vi "XY_plot_gnuplot.vi"(0 "Plot Array":cluster{dbl[], dbl[]}[](array[cluster])=[{[500.0, 500.0, 953.54, 215.0, 270.0, 320.0, 445.0, 525.0, 600.0, 675.0, 750.0, 825.0, 900.0, 960.0, 1010.0, 1060.0], [4.614524, 4.54365, 5.818368, 0.1374656, 0.6662545, 1.465458, 3.619824, 4.848976, 5.887329, 5.940571, 6.152151, 5.717487, 5.600293, 5.40069, 5.154843, 5.121789]}, {[100.0, 150.0, 215.0, 270.0, 320.0, 445.0, 525.0, 600.0, 675.0, 750.0, 825.0, 900.0, 960.0, 1010.0, 1060.0], [0.002314715, -0.00693192, 0.120417, 0.6880509, 1.519176, 3.513709, 5.065183, 6.116033, 6.096773, 5.938465, 5.593788, 5.5597, 5.387002, 5.304077, 4.887903]}] {"?" format="%.2f"; "?" format="%.2f"}, 1 "Job Directory":path=path "/G4_2_HD/Users/paulhayden/Documents/Projects/Westlakes_resolution") -> (2 "Saved Automatically?":bool, 3 "Tex Info String":string="set term epslatex\nset output \"Plot.eps\"\nset xlabel '$Distance~(m)$'\nset ylabel '$DF~(s/m^3)\\times10^6$'\nset samples 1000\nset pointsize 1.00\nset title '$B38~Centreline~Glc$' 0, 0\nset size 0.75,0.9\n\n#set key 450, -2.5833\n unset key\nset label 1 '~~~~~~~~~~~Angle~(deg)~=~0' at -100, -2.58\nset label 2 '~~~~~~~~~~~Height~(m)~=~5' at -100, -3.27\n set xrange [0 : 500] \n# set autoscale x \n set yrange [0.10000 : 7]\n# set autoscale y \n\nplot \"B38_Centreline_Glc.dat\" index 0 using 1:2 axes x1y1 title '$File=B38R~DDD.xls$' with points 1 1, \\\n\"B38_Centreline_Glc.dat\" index 1 using 1:2 axes x1y1 title '$File=B38R~DDD~1.xls$' with points 1 3", 4 "Plot data file":path)   [LabVIEW 2015]
uses:
  Gnuplot_Label.ctl
  gnuplotScriptComponents/gridlines.ctl
  gnuplotScriptComponents/legendAppearance.ctl
  gnuplotScriptComponents/legendProperties.ctl
  gnuplotScriptComponents/alignment.ctl
  gnuplotScriptComponents/at.ctl
  <vilib>/Analysis/baseanly.llb/Mean (DBL).vi
  Results_plotter_Global.vi
  <vilib>/Analysis/NI_AALBase.lvlib
  <vilib>/Analysis/NI_AALPro.lvlib
panel:
  in  "Current Fit Formula":string
  in  "Show Re-Run Gnuplot?":bool
  in  "Tab Control":T1(tab)
  in  "Plot Title":u16(ring) items=["Title String Only", "Stack::", "RunNum::", "WD::(deg)", "EBD::", "Stack:X:(mm ref TTC)", "User:Comments:", "Run:Messages:", "Exclude:Reason:", "X:Rel:(mm)", "Y:Rel:(mm)", "C:minusBG:(ppm)", "C:LatFit:Max(ppm)", "C:LatFit:SigmaY(mm)", "C:LatFit:Yo(mm)", "C:LatData:Max(ppm)", "Uref::(m/s)", "C:incBG:(ppm)", "C:Variance:(ppm^2)", "C:minusBG:(ppm)Err", "C:LatData:Max(ppm)Err", "BG:Conc:(ppm)", "BG:Variance:(ppm^2)", "BG:Conc:(ppm)Err", "FID:Num:", "FID:Calibration:Filename", "X:Trav:(mm)", "Y:Trav:(mm)", "Z (mm)::", "TrackedStack:Yat0deg:(mm)", "TrackedStack:Xat0deg:(mm)", "TrackedStack:Ycurrent:(mm)", "TrackedStack:Xcurrent:(mm)", "T::(C)", "P:Atm:(mbar)", "MFC:Enable:", "MFC24:Read:(%)", "MFC23:Read:(%)", "Date:of:Measurement", "Time:Measurement:Commenced", "Multi Run:Command:Filename", "Multi Run:Start Time:", "Multi Run:Row:Type", "Time:Stamp:(seconds)", "Original:Results:Filename", "Raw:Data:Filename", "EBD:Comments:", "EBD:Xdim:", "EBD:Ydim:", "EBD:Zdim:", "EBD:RunNum:", "EBD:X-Location:", "EBD:Y-Location:", "Number of Measurements"]
  in  "Plot Title":string
  in  "Added labels":i32[](listbox)
  in  "Show Labels?":bool
  in  "Summarise":u16(ring) items=["All Series", "EBD=0L\\times0W\\times0H @  0X, 0Y__Stack X (mm ref TTC)=Show All__", "EBD=80L\\times160W\\times80H @  -80X, 0Y__Stack X (mm ref TTC)=Show All__", "EBD=80L\\times160W\\times80H @  0X, 0Y__Stack X (mm ref TTC)=Show All__", "EBD=90L\\times180W\\times90H @  0X, 0Y__Stack X (mm ref TTC)=Show All__", "EBD=100L\\times200W\\times100H @  -100X, 0Y__Stack X (mm ref TTC)=Show All__"]
  in  "X Log?":bool
  in  "Y Log?":bool
  in  "Ymin Val":dbl
  in  "Ymin":bool=TRUE
  in  "Xmin Val":dbl
  in  "Xmin":bool=TRUE
  in  "Xmax Val":dbl
  in  "Xmax":bool=TRUE
  in  "Ymax Val":dbl
  in  "Ymax":bool=TRUE
  in  "Major Gridlines":T2
  in  "Minor Gridlines":T2
  out "Time format?":bool
  in  "precision":string
  out "Profile offset":dbl
  in  "Offset?":bool
  in  "Mode":T3
  in  "Separation":dbl=1.2
  in  "Fit Line Width":i32=2
  in  "Fit type":T4(ring)
  in  "Put Coeff\nin Results file":bool
  in  "Analysis":T5(ring)
  in  "Wavelength?":bool
  in  "Auto Zp":bool=TRUE
  in  "Fixed Zp":dbl format="%.2f"
  in  "Something about fit..!":bool
  in  "Fit Line Type":i32=2
  in  "Black and white?":bool
  in  "plot error bars?":bool
  in  "Plot style":u16[](array[ring])=[0, 0, 0, 0, 0, 0, 0, 0, 0, 0, 0] items=["points", "lines", "linespoints"]
  in  "Point Size":dbl=1.2 format="%.2f"
  in  "Graph Height":string="0.9"
  in  "Graph width":string="0.75"
  in  "Reverse order":bool
  in  "Appearance":T6
  in  "Show legend?":bool
  in  "Legend Position":u16(ring) items=["LabVIEW calculated", "top left", "top right", "bottom left", "bottom right", "below"]
  in  "Save data analysis file":bool
  out "Path":path
  in  "Filename Max length":i32=28
  out "With legend":i32=580
  out "No Legend":i32=397
  out "No of Series":i32=2
  out "X location":dbl=-100.0
  out "Y location":dbl=-2.583333333333333
  out "Delta y":dbl=0.6900000000000001
  out "Extra range":dbl
  out "Final Title":string="B38 Centreline Glc"
  out "XY Graph":cluster{dbl[], dbl[]}[](graph)=[{[215.0, 270.0, 320.0, 445.0, 500.0, 500.0, 525.0, 600.0, 675.0, 750.0, 825.0, 900.0, 953.54, 960.0, 1010.0, 1060.0], [0.1374656, 0.6662545, 1.465458, 3.619824, 4.614524, 4.54365, 4.848976, 5.887329, 5.940571, 6.152151, 5.717487, 5.600293, 5.818368, 5.40069, 5.154843, 5.121789]}, {[100.0, 150.0, 215.0, 270.0, 320.0, 445.0, 525.0, 600.0, 675.0, 750.0, 825.0, 900.0, 960.0, 1010.0, 1060.0], [0.002314715, -0.00693192, 0.120417, 0.6880509, 1.519176, 3.513709, 5.065183, 6.116033, 6.096773, 5.938465, 5.593788, 5.5597, 5.387002, 5.304077, 4.887903]}]
  # "Scales"
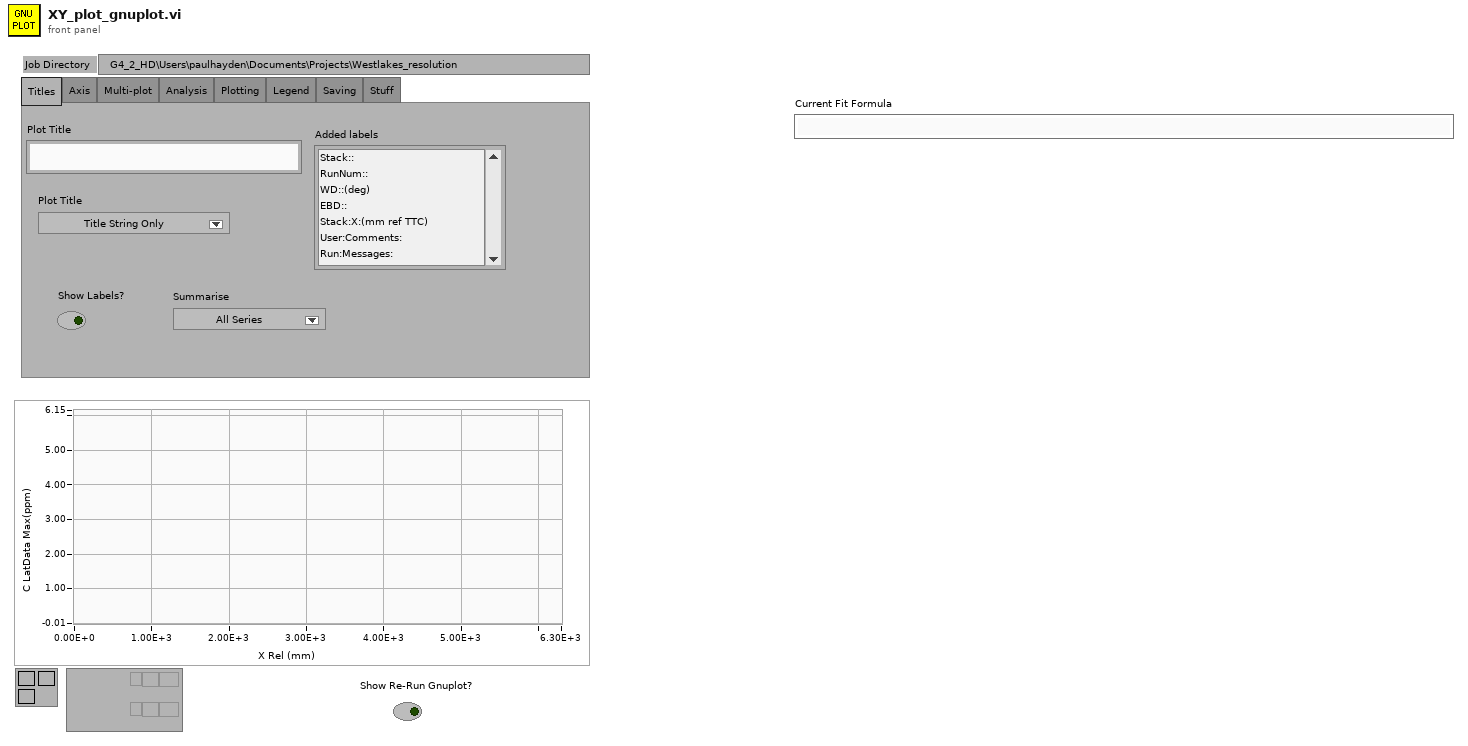
[diagram p1: front panel]
types:
  T1 = enum32{"Titles", "Axis", "Multi-plot", "Analysis", "Plotting", "Legend", "Saving", "Stuff"}
  T2 = typedef "gridlines.ctl" = enum16{"None", "X only", "Y only", "Both X and Y"}
  T3 = typedef "Gnuplot_Label.ctl" = enum16{"3 Labels per plot", "Only Center label", "Only Bottom Label"}
  T4 = enum16{"None", "Spline", "Linear", "2nd Poly", "3rd Poly", "4th Poly", "Gauss Lat", "Gauss vert", "Gauss Vert with 2 sig", "Guass glc"}
  T5 = enum16{"None", "% change", "Spectrum", "Norm Spec"}
  T6 = typedef "legendAppearance.ctl" = cluster{"layout":string, "text-sample order":string, "key order":string, "surroundingBox":string, "MaxRows":u32, "MaxCols":u32, "WidthAdjust":dbl}
  T7 = cluster{"Output":dbl[], "PercentageDifferenceArray":dbl[]}[]
  T8 = cluster{"Output":dbl[], "PercentageDifferenceArray":dbl[]}
  T9 = typedef "legendProperties.ctl" = cluster{"Appearance":T6, "Alignment":T10, "Location":string, "\"At\" location":T11}
  T10 = typedef "alignment.ctl" = cluster{"Horizontal":string, "Vertical":string}
  T11 = typedef "at.ctl" = cluster{"XcoordSys":string, "YcoordSys":string, "Xvalue":dbl, "Yvalue":dbl}
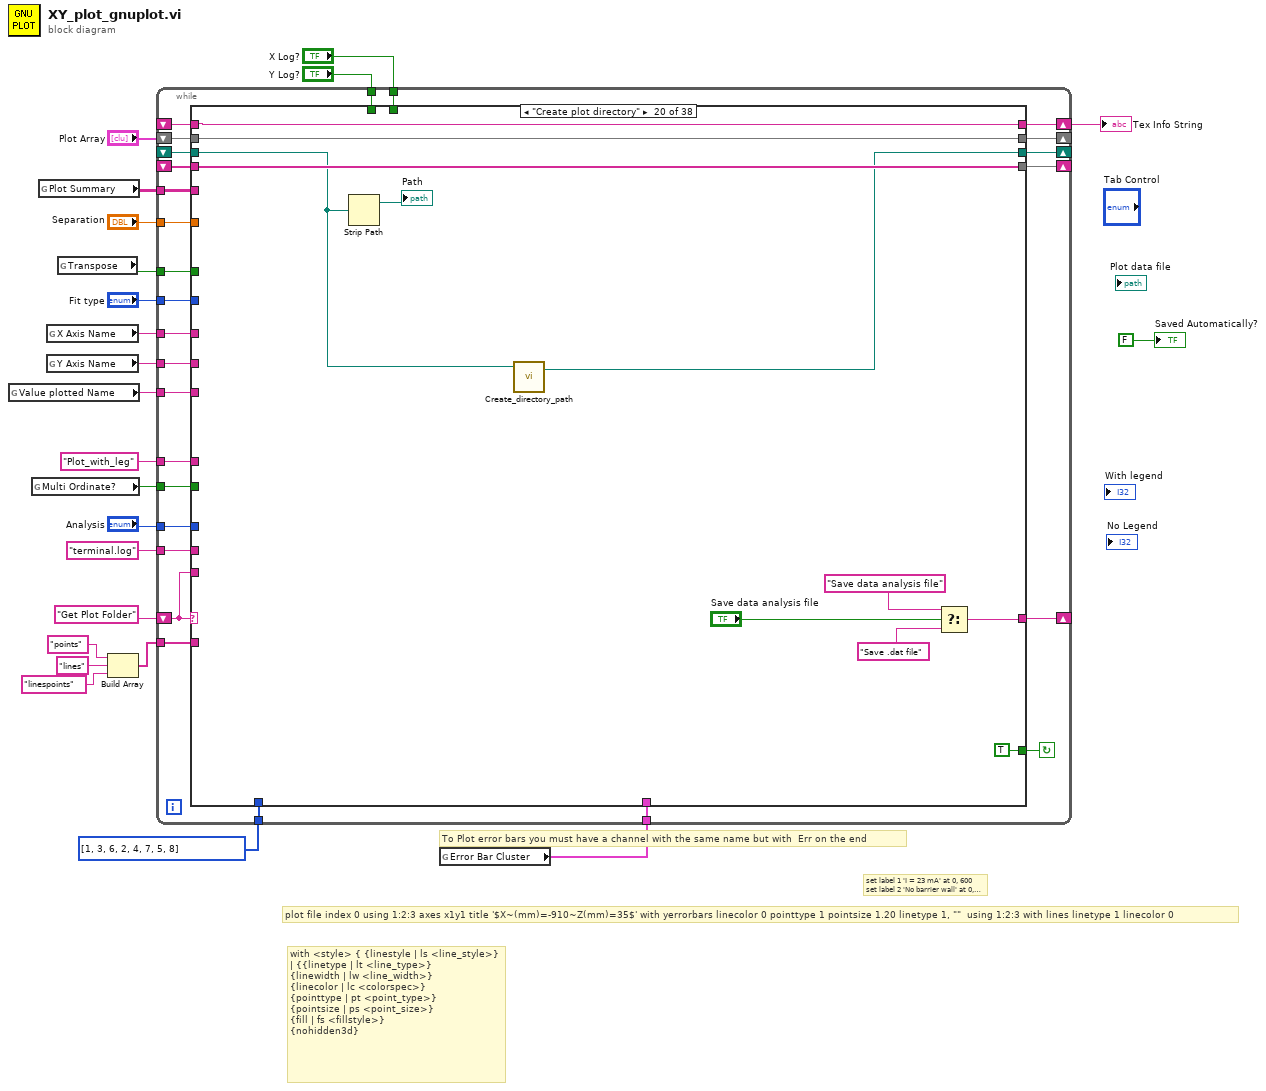
[diagram p0: block diagram]
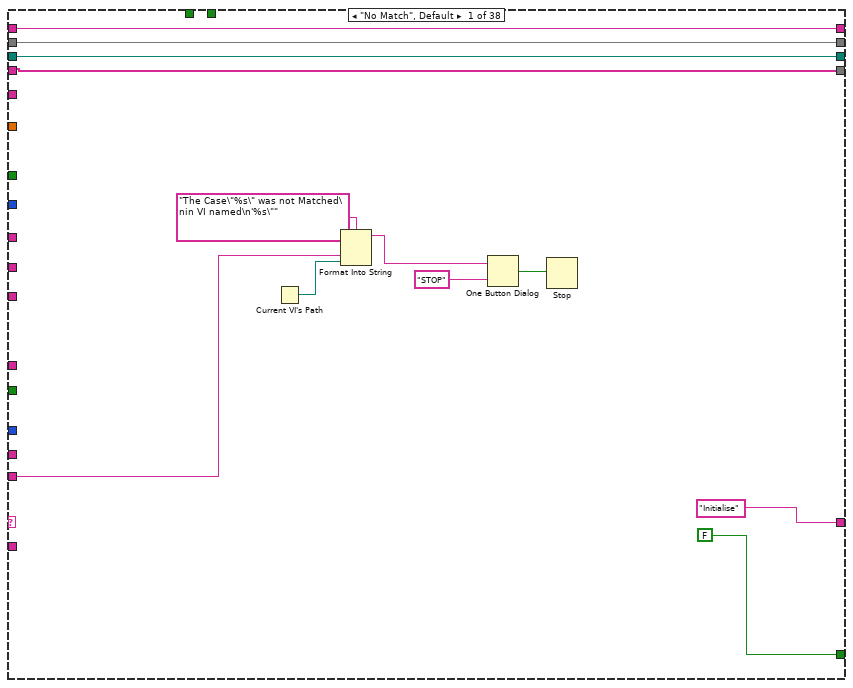
[diagram p2: hidden frame]
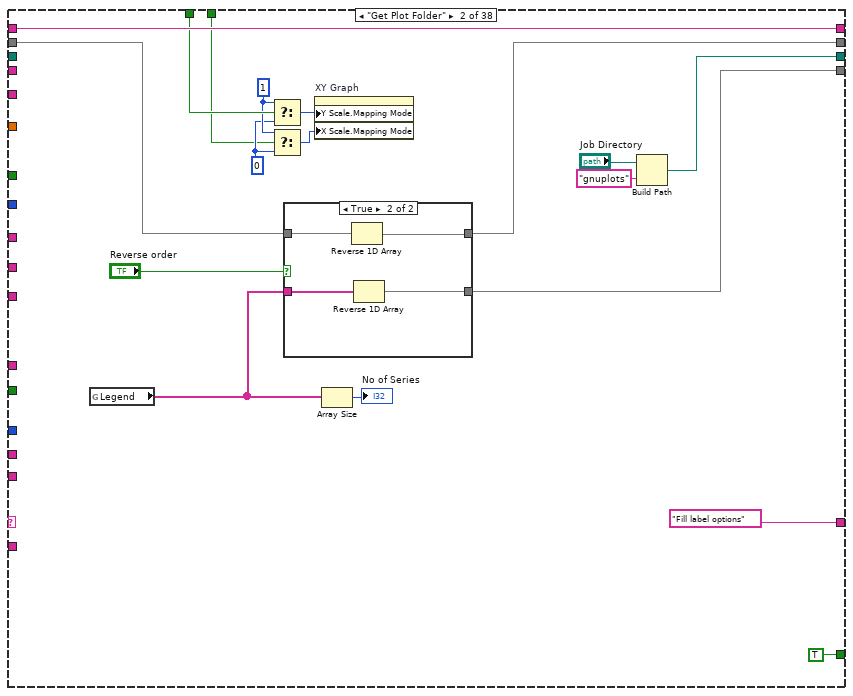
[diagram p3: hidden frame]
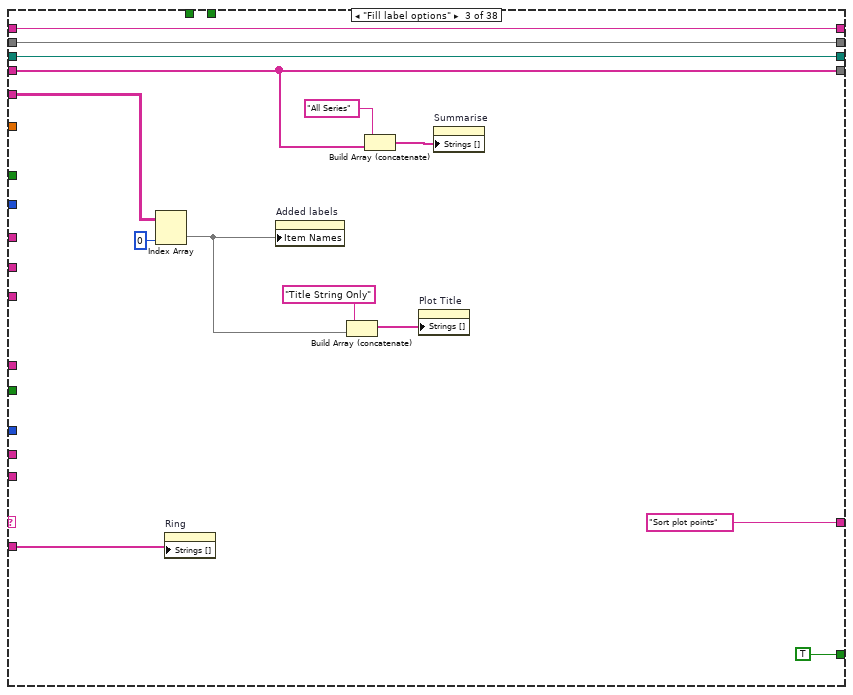
[diagram p5: hidden frame]
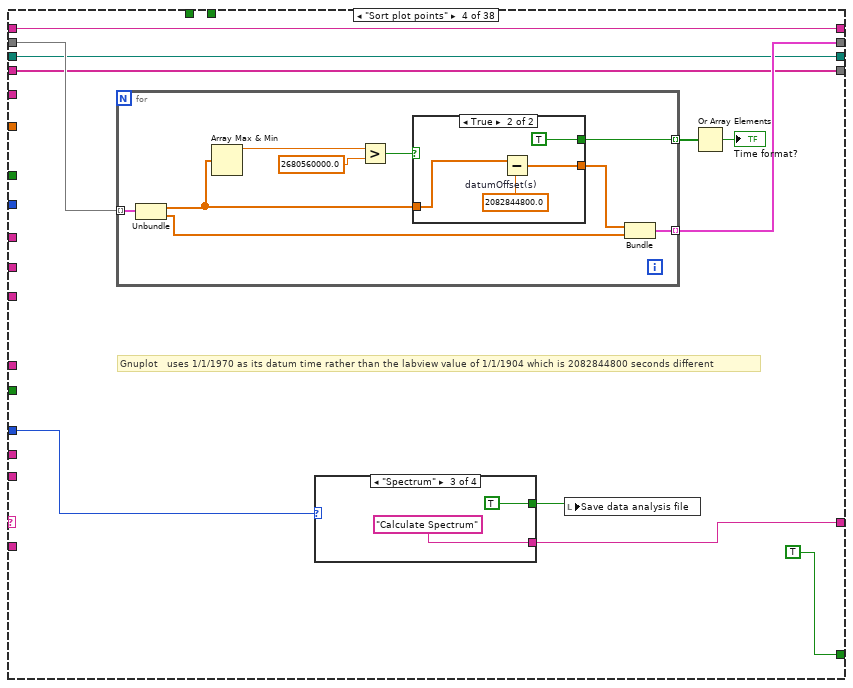
[diagram p6: hidden frame]
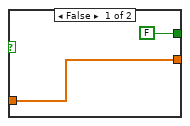
[diagram p7: hidden frame]
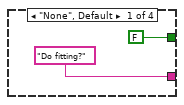
[diagram p8: hidden frame]
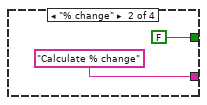
[diagram p9: hidden frame]
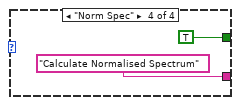
[diagram p10: hidden frame]
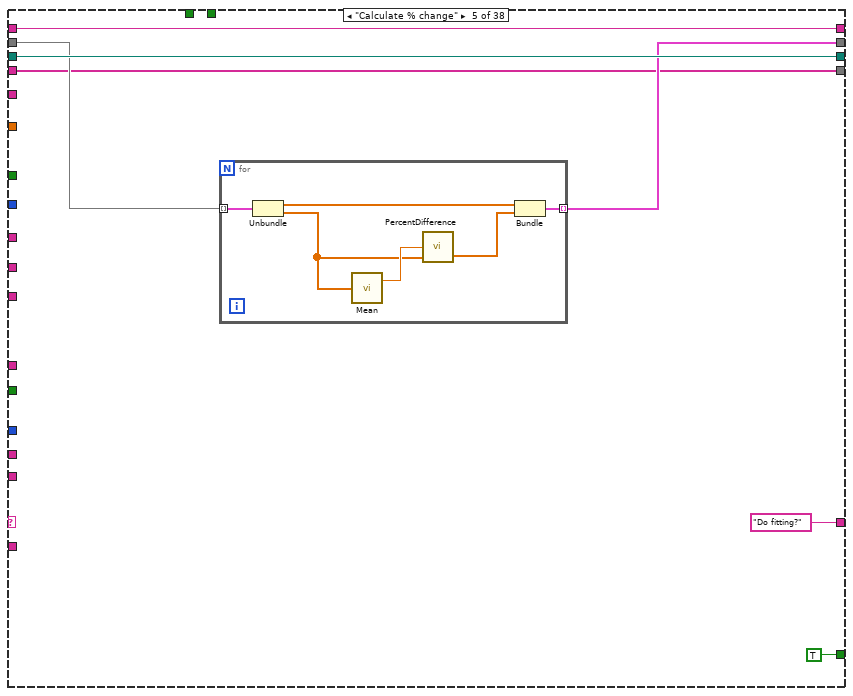
[diagram p11: hidden frame]
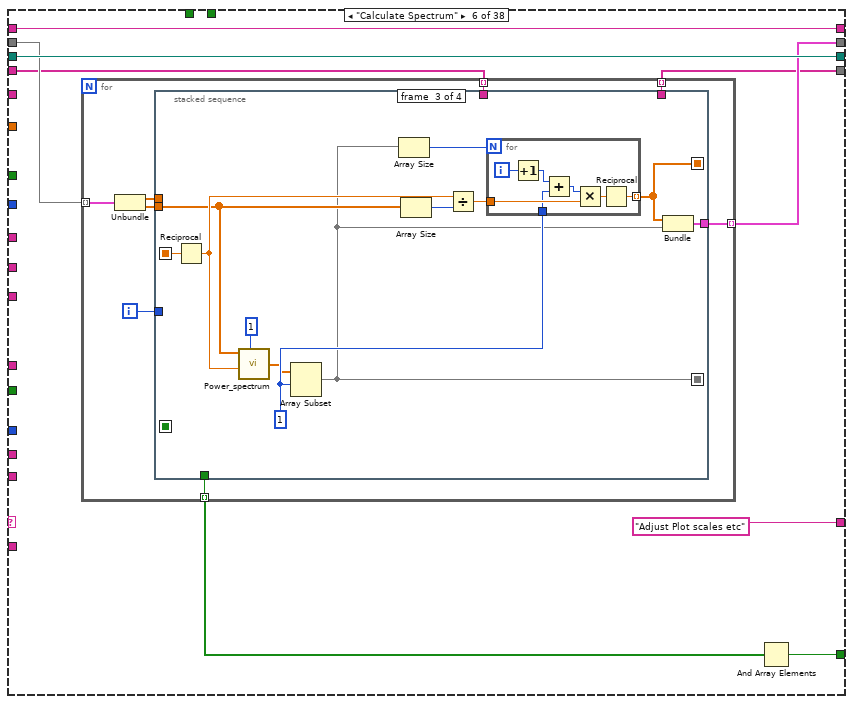
[diagram p12: hidden frame]
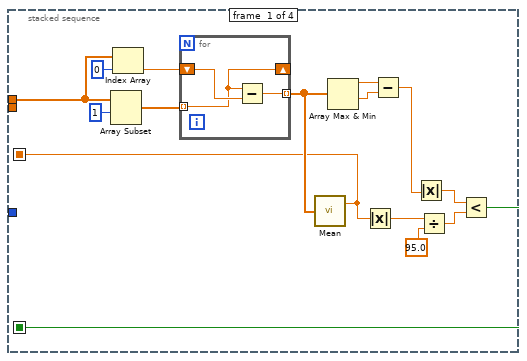
[diagram p13: hidden frame]
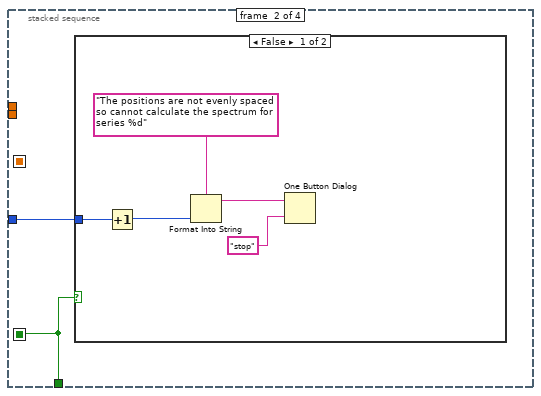
[diagram p14: hidden frame]
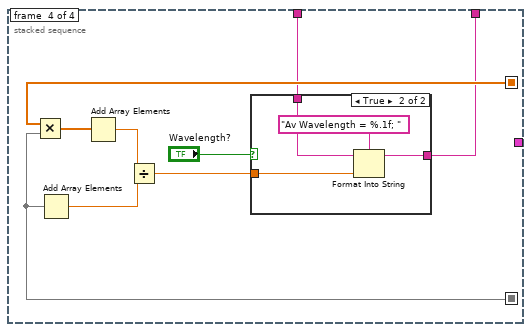
[diagram p16: hidden frame]
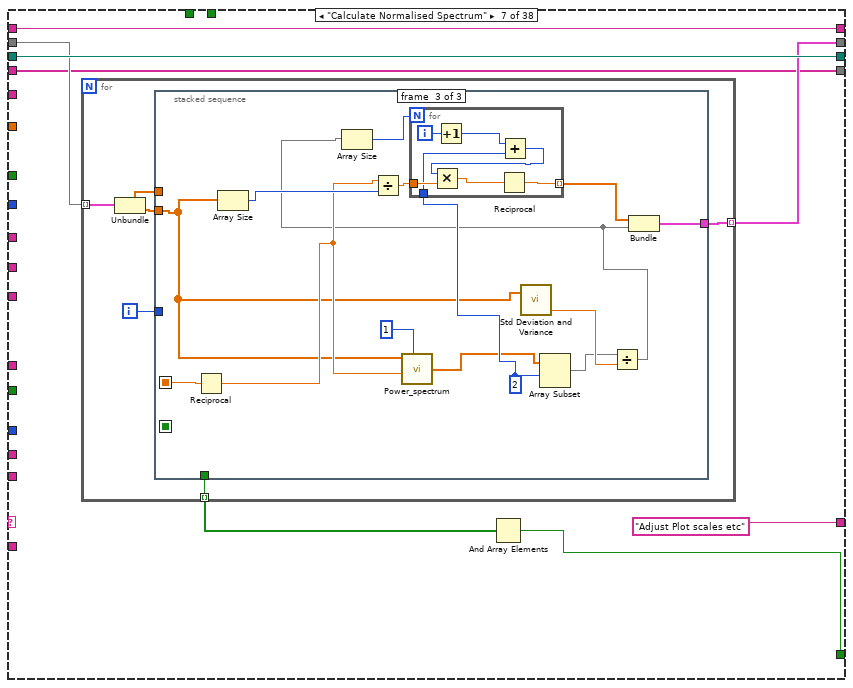
[diagram p18: hidden frame]
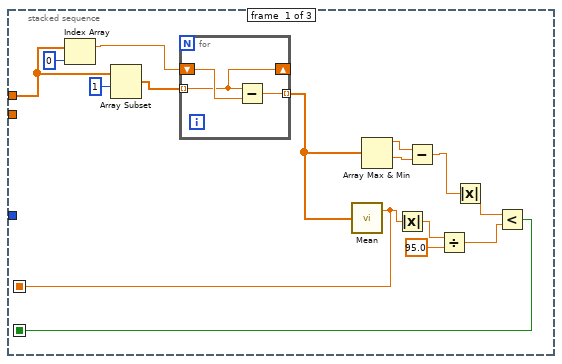
[diagram p19: hidden frame]
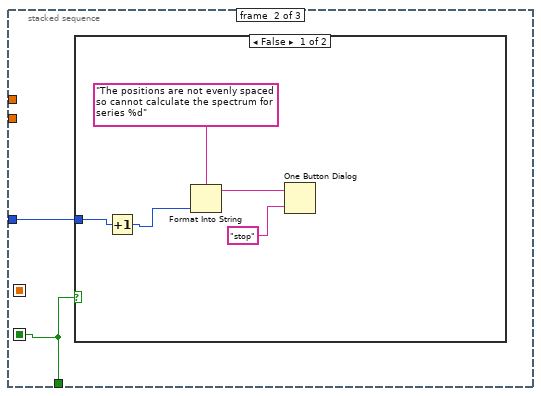
[diagram p20: hidden frame]
diagram:
  # "plot file index 0 using 1:2:3 axes x1y1 title '$X~(mm)=-910~Z(mm)=35$' with yerrorbars linecolor 0 pointtype 1 pointsize 1.20 linetype 1, \"\"  using 1:2:3 with lines linetype 1 linecolor 0"
  # "with <style> { {linestyle | ls <line_style>} \n| {{linetype | lt <line_type>} \n{linewidth | lw <line_width>} \n{linecolor | lc <colorspec>} \n{pointtype | pt <point_type>} \n{pointsize | ps <point_size>} \n{fill | fs <fillstyle>} \n{nohidden3d}"
  # "To Plot error bars you must have a channel with the same name but with  Err on the end"
  # "set label 1 'I = 23 mA' at 0, 600\nset label 2 'No barrier wall' at 0, 300"
  n1 = global read "Results_plotter_Global.vi" "Value plotted Name"() -> (w19:string)
  n2 = global read "Results_plotter_Global.vi" "Multi Ordinate?"() -> (w1:bool)
  n3 = global read "Results_plotter_Global.vi" "Plot Summary"() -> (w22:string[][])
  n4 = global read "Results_plotter_Global.vi" "X Axis Name"() -> (w21:string)
  n5 = global read "Results_plotter_Global.vi" "Y Axis Name"() -> (w20:string)
  n6 = global read "Results_plotter_Global.vi" "Transpose"() -> (w2:bool)
  n7 = Build Array("points", "lines", "linespoints") -> (w9:string[])
  n8 = global read "Results_plotter_Global.vi" "Error Bar Cluster"() -> (w4:cluster{string[]}[])
  n9 = while {
    shift-left: "Get Plot Folder" -> [w48]
    shift-right: [w49] -> _
    tunnel: w22 -> [w47]
    shift-right: [w46] -> _
    shift-left: _ -> [w45]
    tunnel: "Analysis" -> [w44]
    tunnel: w21 -> [w43]
    tunnel: w20 -> [w42]
    tunnel: w19 -> [w41]
    shift-right: [w39] -> _
    shift-left: "Plot Array" -> [w40]
    shift-right: [w37] -> w17
    shift-left: _ -> [w38]
    tunnel: "Plot_with_leg" ("name or relative path") -> [w36]
    tunnel: "Fit type" -> [w35]
    shift-right: [w34] -> _
    shift-left: _ -> [w33]
    tunnel: "terminal.log" -> [w32]
    tunnel: w9 -> [w31]
    tunnel: i32[] [1, 3, 6, 2, 4, 7, 5, 8] ("Plot style") -> [w30]
    tunnel: "Separation" -> [w29]
    tunnel: "Y Log?" -> [w28]
    tunnel: w4 -> [w27]
    tunnel: "X Log?" -> [w26]
    tunnel: w2 -> [w25]
    tunnel: w1 -> [w24]
    stop <- w50 continue-if-true
    n10 = case shown="\"Create plot directory\"" w48 {
      tunnel: [FALSE TRUE TRUE ("Top Level") TRUE TRUE w150 w223 TRUE TRUE TRUE ("Top Level") TRUE ("Top Level") TRUE ("Top Level") TRUE ("Top Level") TRUE ("Top Level") TRUE ("Top Level") TRUE ("Top Level") TRUE ("Top Level") TRUE ("Top Level") TRUE ("Top Level") TRUE ("Top Level") w672 w745 TRUE ("Top Level") TRUE ("Top Level") TRUE ("Top Level") TRUE ("Top Level") TRUE ("Top Level") TRUE ("Top Level") TRUE ("Top Level") TRUE ("Top Level") TRUE ("Top Level") TRUE ("Top Level") TRUE ("Top Level") TRUE ("Top Level") TRUE ("Top Level") w1576 FALSE ("Top Level") FALSE ("Top Level")] -> w50
      tunnel: ["Initialise" "Fill label options" "Sort plot points" w104 "Do fitting?" "Adjust Plot scales etc" "Adjust Plot scales etc" "Adjust Plot scales etc" "Add fitted line styles" "Adjust Plot scales etc" w379 "Fill Second legend" "Fill Second legend" "Fill Second legend" "Calculate plot max and min values" "Sort out plot title" w564 w634 "Create plot directory" w658 w671 w744 w888 "Edit Legend names" w1076 "Labels?" ("t") "Labels?" ("t") w1239 w1250 "Plot Command" "Write gnuplot file" ("t") "Execute shell script" ("t") "Has pdf been generated?" ("t") w1552 "Input Fit Coefficients into results file?" "Read Fit Coefficients" ("t") "End" ("t") "End" ("t")] -> w49
      tunnel: w48 -> [w57 _ _ _ _ _ _ _ _ _ _ _ _ _ _ _ _ _ _ _ _ _ _ _ _ _ _ _ _ _ _ _ _ _ _ _ _ _]
      tunnel: w47 -> [_ _ w100 _ _ _ _ _ _ _ _ _ _ _ _ _ w573 _ _ _ w670 w743 _ _ _ _ _ _ w1249 _ _ _ _ _ _ _ _ _]
      tunnel: [w54 w77 w94 w108 w139 w155 w229 w288 w303 w364 w389 w415 w424 w436 w463 w497 w566 w635 w646 w660 w673 w746 w900 w942 w1091 w1159 w1216 w1246 w1256 w1382 w1414 w1537 w1545 w1558 w1569 w1580 w1598 w1725] -> w46
      tunnel: w45 -> [w54 _ w94 w108 w139 w155 w229 w288 w303 w364 w389 w415 w424 w436 w459 w497 w565 w631 w647 w655 w673 w746 w900 w942 w1091 w1159 w1216 w1246 w1256 w1382 w1414 w1537 w1545 w1558 w1569 w1580 w1598 w1725]
      tunnel: w44 -> [_ _ _ w105 _ _ _ _ _ _ w380 _ _ w430 _ _ _ w622 _ _ w666 w738 w897 _ _ _ _ _ _ _ _ _ _ _ _ _ _ _]
      tunnel: w43 -> [_ _ _ _ _ _ _ _ w294 _ _ w411 w423 _ _ _ _ _ _ _ w669 w742 w895 _ _ _ _ _ _ _ _ _ _ _ _ _ _ _]
      tunnel: w42 -> [_ _ _ _ _ _ _ _ w293 _ _ w410 w422 w435 _ _ _ _ _ _ w668 w741 w896 _ _ _ _ _ _ _ _ _ _ _ _ _ _ _]
      tunnel: w41 -> [_ _ _ _ _ _ _ _ _ _ _ _ _ _ _ _ _ _ _ _ w665 _ _ _ _ _ _ _ _ _ _ _ _ _ _ _ w1586 _]
      tunnel: w40 -> [w53 w72 w95 w110 w138 w154 w228 w284 w299 w363 w378 w414 w421 w434 w462 w494 w579 w633 w650 w663 w664 w740 w901 w930 w1086 w1154 w1212 w1243 w1251 w1383 w1415 w1543 w1550 w1565 w1574 w1584 w1591 w1730]
      tunnel: [w53 w71 w95 w109 w137 w153 w227 w284 w292 w363 w378 w414 w421 w434 w462 w494 w579 w633 w650 w663 w664 w737 w901 w930 w1086 w1154 w1212 w1243 w1251 w1383 w1415 w1543 w1550 w1565 w1574 w1584 w1591 w1730] -> w39
      tunnel: w38 -> [w52 w76 w96 w107 w136 w152 w226 w287 w302 w361 w381 w413 w420 w433 w461 w498 w574 w632 w649 w662 w674 w747 _ w940 w1090 w1125 w1192 w1234 w1253 w1380 w1412 w1532 w1548 w1563 w1572 w1582 w1601 w1728]
      tunnel: [w52 w76 w96 w107 w136 w152 w226 w287 w302 w361 w381 w413 w420 w433 w461 w498 w574 w632 w649 w662 w674 w747 w891 w938 w1090 w1122 w1191 w1233 w1254 w1376 w1411 w1532 w1548 w1563 w1572 w1582 w1601 w1728] -> w37
      tunnel: w36 -> [_ _ _ _ _ _ _ _ _ _ _ _ _ _ _ _ _ _ _ _ _ _ _ _ _ _ _ _ _ _ _ _ _ _ _ _ _ _]
      tunnel: w35 -> [_ _ _ _ _ _ _ w285 w301 _ w383 _ _ _ _ _ _ _ _ _ _ _ w889 w944 _ _ _ _ _ w1349 w1408 _ _ _ _ w1579 w1594 _]
      tunnel: [w51 w70 w92 w106 w135 w148 w225 w286 w296 w360 w385 w412 w419 w432 w460 w496 w578 w630 w648 w661 w667 w739 w899 w945 w1092 w1158 w1215 w1245 w1255 w1370 w1413 w1538 w1549 w1564 w1573 w1583 w1602 w1729] -> w34
      tunnel: w33 -> [w51 _ w92 w106 w135 w149 w225 w286 w297 w360 w385 w412 w419 w432 w460 w496 w578 w630 w648 w661 w667 w739 w899 w945 w1093 w1158 w1215 w1245 w1255 w1370 w1413 w1538 w1549 w1564 w1573 w1583 w1602 w1729]
      tunnel: w32 -> [_ _ _ _ _ _ _ _ _ _ _ _ _ _ _ _ _ _ _ _ _ _ _ _ _ _ _ _ _ _ _ _ w1544 _ _ _ _ w1723]
      tunnel: w31 -> [_ _ w90 _ _ _ _ _ _ _ _ _ _ _ _ _ _ _ _ _ _ _ _ _ _ _ _ _ _ _ _ _ _ _ _ _ _ _]
      tunnel: w30 -> [_ _ _ _ _ _ _ _ _ _ _ _ _ _ _ _ _ _ _ _ _ _ _ _ _ _ _ _ _ _ w1406 w1534 _ _ _ _ _ _]
      tunnel: w29 -> [_ _ _ _ _ _ _ _ _ _ _ _ _ _ _ _ _ _ _ _ _ w736 _ _ w1085 _ _ _ _ w1367 _ _ _ _ _ _ _ _]
      tunnel: w28 -> [_ w69 _ _ _ _ _ _ _ _ _ _ _ _ _ _ _ _ _ _ _ _ _ _ _ w1138 w1203 _ w1248 w1364 _ _ _ _ _ _ _ _]
      tunnel: w27 -> [_ _ _ _ _ _ _ _ _ _ _ _ _ _ _ w467 _ _ _ _ _ w735 _ _ _ _ _ _ _ _ w1405 _ _ _ _ _ _ _]
      tunnel: w26 -> [_ w64 _ _ _ _ _ _ _ _ _ _ _ _ _ _ _ _ _ _ _ _ _ _ _ w1135 _ _ w1247 w1359 _ _ _ _ _ _ _ _]
      tunnel: w25 -> [_ _ _ _ _ _ _ _ _ _ _ _ _ _ _ w465 _ _ _ _ _ w734 _ w931 _ _ _ _ _ w1354 w1402 _ _ _ _ _ _ _]
      tunnel: w24 -> [_ _ _ _ _ _ _ _ _ _ _ _ _ _ _ _ _ _ _ _ _ _ _ _ _ _ _ _ _ _ _ _ _ _ _ _ _ _]
      frame "No Match", Default {
        n11 = Current VI's Path() -> (path=w56:path)
        n12 = Format Into String(format string="The Case\"%s\" was not Matched\nin VI named\n'%s\"" ("Format String"), w57, w56) -> (resulting string=w60:string)  [unwired: 2 in, 1 out]
        n13 = One Button Dialog(message=w60, button name ("OK")="STOP") -> (true=w58:bool)
        n14 = Stop(stop? (T)=w58) -> ()
      }
      frame "Get Plot Folder" {
        w65 = u8 0 ("f")
        w66 = u8 1 ("Y Scale.Mapping Mode")
        n15 = global read "Results_plotter_Global.vi" "Legend"() -> (w63:string[])
        n16 = Select(t=w66, s=w69, f=w65) -> (s? t:f=w68:u8)
        n17 = Select(t=w66, s=w64, f=w65) -> (s? t:f=w67:u8)
        n18 = case shown="True" "Reverse order" {
          tunnel: w72 -> [w82 w86]
          tunnel: [w82 w85] -> w71
          tunnel: w63 -> [w81 w84]
          tunnel: [w81 w83] -> w70
          frame False {
          }
          frame True {
            n19 = Reverse 1D Array(array=w86) -> (reversed array=w85:T7)
            n20 = Reverse 1D Array(array=w84) -> (reversed array=w83:string[])
          }
        }
        n21 = property on="XY Graph" class="XYGraph (strict)"("Y Scale.Mapping Mode"=w68, "X Scale.Mapping Mode"=w67) -> ()  [unwired: 2 in, 2 out]
        n22 = Array Size(array=w63) -> (size(s)=→"No of Series":i32)
        n23 = Build Path(base path="Job Directory", name or relative path="gnuplots") -> (appended path=w77:path)
      }
      frame "Fill label options" {
        n24 = Index Array(array=w100, index (col)=0 ("disabled index (col)")) -> (element=w88:string[])  [unwired: 1 in]
        n25 = property on="Ring" class="Ring (strict)"("Strings []"=w90) -> ()  [unwired: 2 in, 2 out]
        n26 = property on="Added labels" class="LstBox (strict)"("Item Names"=w88) -> ()  [unwired: 2 in, 2 out]
        n27 = Build Array (concatenate)("Title String Only", w88) -> (w87:string[])
        n28 = Build Array (concatenate)("All Series", w92) -> (w93:string[])
        n29 = property on="Plot Title" class="Ring (strict)"("Strings []"=w87) -> ()  [unwired: 2 in, 2 out]
        n30 = property on="Summarise" class="Ring (strict)"("Strings []"=w93) -> ()  [unwired: 2 in, 2 out]
      }
      frame "Sort plot points" {
        # "Gnuplot   uses 1/1/1970 as its datum time rather than the labview value of 1/1/1904 which is 2082844800 seconds different"
        n31 = for {
          tunnel: w110 -> [w119] mode=indexing
          tunnel: [w120] -> w109 mode=indexing
          tunnel: [w112] -> w102 mode=indexing
          n32 = Unbundle(w119) -> ("Output"=w115:dbl[], "PercentageDifferenceArray"=w116:dbl[])
          n33 = Array Max & Min(array=w115) -> (max value=w118:dbl)  [unwired: 3 out]
          n34 = Greater?(x=w118, y=2680560000.0) -> (0:w113:bool)
          n35 = case shown="True" w113 {
            tunnel: w115 -> [w122 w126]
            tunnel: [w122 w124] -> w114
            tunnel: [FALSE TRUE] -> w112
            frame False {
            }
            frame True {
              w125 = 2082844800.0  # datumOffset(s)
              n36 = Subtract(x=w126, y=w125) -> (x-y=w124:dbl[])
            }
          }
          n37 = Bundle("Output"=w114, "PercentageDifferenceArray"=w116) -> (w120:T8)  [unwired: 1 out]
        }
        n38 = case shown="\"Spectrum\"" w105 {
          tunnel: ["Do fitting?" "Calculate % change" "Calculate Spectrum" "Calculate Normalised Spectrum"] -> w104
          tunnel: [FALSE ("Save data analysis file") FALSE ("Save data analysis file") TRUE ("Save data analysis file") TRUE ("Save data analysis file")] -> w103
          frame "None", Default {
          }
          frame "% change" {
          }
          frame "Spectrum" {
          }
          frame "Norm Spec" {
          }
        }
        n39 = local write "Save data analysis file"(w103) -> ()
        n40 = Or Array Elements(Boolean array=w102) -> (logical OR=→"Time format?":bool)
      }
      frame "Calculate % change" {
        n41 = for {
          tunnel: w138 -> [w147] mode=indexing
          tunnel: [w145] -> w137 mode=indexing
          n42 = Unbundle(w147) -> ("Output"=w146:dbl[], "PercentageDifferenceArray"=w143:dbl[])
          n43 = call-poly <vilib>:"Mean.vi"("X"=w143) -> ("mean"=w144:dbl)  [unwired: 1 out]
          n44 = call "PercentDifference.vi"("CompareeArray"=w143, "Basis"=w144) -> ("PercentageDifferenceArray"=w142:dbl[])  [unwired: 1 in, 1 out]
          n45 = Bundle("Output"=w146, "PercentageDifferenceArray"=w142) -> (w145:T8)  [unwired: 1 out]
        }
      }
      frame "Calculate Spectrum" {
        n46 = for {
          tunnel: w154 -> [w163] mode=indexing
          tunnel: [w164] -> w153 mode=indexing
          tunnel: [w159] -> w151 mode=indexing
          tunnel: w149 -> [w158] mode=indexing
          tunnel: [w157] -> w148 mode=indexing
          i -> [w160]
          n47 = Unbundle(w163) -> ("Output"=w161:dbl[], "PercentageDifferenceArray"=w162:dbl[])
          n48 = stacked-sequence {
            seq-local: [w166 _ _ _] -> [_ _ w196 _]
            seq-local: [w165 _ _ _] -> [_ w183 _ _]
            seq-local: [_ _ w192 _] -> [_ _ _ w216]
            seq-local: [_ _ w191 _] -> [_ _ _ w217]
            tunnel: [_ _ w201 _] -> w164
            tunnel: w162 -> [_ _ w194 _]
            tunnel: w161 -> [w177 _ _ _]
            tunnel: w160 -> [_ w184 _ _]
            tunnel: [_ w183 _ _] -> w159
            tunnel: w158 -> [_ _ _ w212]
            tunnel: [_ _ _ w210] -> w157
            frame #0 {
              n49 = Array Subset(array=w177, index=1) -> (w175:dbl[])  [unwired: 1 in]
              n50 = Index Array(array=w177, index=0) -> (element=w176:dbl)
              n51 = for {
                shift-right: [w181] -> _
                shift-left: w176 -> [w182]
                tunnel: w175 -> [w181] mode=indexing
                tunnel: [w180] -> w172 mode=indexing
                n52 = Subtract(x=w181, y=w182) -> (x-y=w180:dbl)
              }
              n53 = call-poly <vilib>:"Mean.vi"("X"=w172) -> ("mean"=w166:dbl)  [unwired: 1 out]
              n54 = Array Max & Min(array=w172) -> (max value=w174:dbl, min value=w173:dbl)  [unwired: 2 out]
              n55 = Absolute Value(x=w166) -> (abs(x)=w169:dbl)
              n56 = Subtract(x=w174, y=w173) -> (x-y=w171:dbl)
              n57 = Absolute Value(x=w171) -> (abs(x)=w170:dbl)
              n58 = Divide(x=w169, y=95.0) -> (x/y=w167:dbl)
              n59 = Less?(x=w170, y=w167) -> (x < y?=w165:bool)
            }
            frame #1 {
              n60 = case shown="False" w183 {
                tunnel: w184 -> [w189 _]
                frame False {
                  n61 = Increment(x=w189) -> (x+1=w188:i32)
                  n62 = Format Into String(format string="The positions are not evenly spaced so cannot calculate the spectrum for series %d", w188) -> (resulting string=w186:string)  [unwired: 2 in, 1 out]
                  n63 = One Button Dialog(message=w186, button name ("OK")="stop") -> ()  [unwired: 1 out]
                }
                frame True {
                }
              }
            }
            frame #2 {
              w197 = 1 ("index")
              n64 = Reciprocal(x=w196) -> (1/x=w195:dbl)
              n65 = call "Power_spectrum.vi"("U"=w194, "Sampling frequency"=w195, "Block No"=1) -> ("SingleBlockSpectrum"=w190:dbl[])  [unwired: 2 in, 2 out]
              n66 = Array Subset(array=w190, index=w197) -> (w191:dbl[])  [unwired: 1 in]
              n67 = Array Size(array=w191) -> (size(s)=w200:i32)
              n68 = Array Size(array=w194) -> (size(s)=w198:i32)
              n69 = Divide(x=w195, y=w198) -> (x/y=w193:dbl)
              n70 = for {
                N: w200 -> [_]
                tunnel: [w205] -> w192 mode=indexing
                tunnel: w193 -> [w207]
                tunnel: w197 -> [w203]
                i -> [w208]
                n71 = Increment(x=w208) -> (x+1=w204:i32)
                n72 = Add(x=w204, y=w203) -> (x+y=w202:i32)
                n73 = Multiply(x=w202, y=w207) -> (x*y=w206:dbl)
                n74 = Reciprocal(x=w206) -> (1/x=w205:dbl)
              }
              n75 = Bundle(w192, w191) -> (w201:cluster{dbl[], dbl[]})  [unwired: 1 out]
            }
            frame #3 {
              n76 = Multiply(x=w216, y=w217) -> (x*y=w215:dbl[])
              n77 = Add Array Elements(numeric array=w217) -> (sum=w213:dbl)
              n78 = Add Array Elements(numeric array=w215) -> (sum=w214:dbl)
              n79 = Divide(x=w214, y=w213) -> (x/y=w211:dbl)
              n80 = case shown="True" "Wavelength?" {
                tunnel: w212 -> [w218 w222]
                tunnel: w211 -> [_ w221]
                tunnel: [w218 w219] -> w210
                frame False {
                }
                frame True {
                  n81 = Format Into String(format string="Av Wavelength = %.1f; ", initial string=w222, w221) -> (resulting string=w219:string)  [unwired: 1 in, 1 out]
                }
              }
            }
          }
        }
        n82 = And Array Elements(Boolean array=w151) -> (logical AND=w150:bool)
      }
      frame "Calculate Normalised Spectrum" {
        n83 = for {
          tunnel: w228 -> [w235] mode=indexing
          tunnel: [w236] -> w227 mode=indexing
          tunnel: [w231] -> w224 mode=indexing
          i -> [w232]
          n84 = Unbundle(w235) -> ("Output"=w233:dbl[], "PercentageDifferenceArray"=w234:dbl[])
          n85 = stacked-sequence {
            seq-local: [w238 _ _] -> [_ _ w269]
            seq-local: [w237 _ _] -> [_ w255 _]
            tunnel: [_ _ w275] -> w236
            tunnel: w234 -> [_ _ w267]
            tunnel: w233 -> [w249 _ _]
            tunnel: w232 -> [_ w256 _]
            tunnel: [_ w255 _] -> w231
            frame #0 {
              n86 = Index Array(array=w249, index=0) -> (element=w248:dbl)
              n87 = Array Subset(array=w249, index=1) -> (w247:dbl[])  [unwired: 1 in]
              n88 = for {
                shift-right: [w253] -> _
                shift-left: w248 -> [w254]
                tunnel: w247 -> [w253] mode=indexing
                tunnel: [w252] -> w244 mode=indexing
                n89 = Subtract(x=w253, y=w254) -> (x-y=w252:dbl)
              }
              n90 = call-poly <vilib>:"Mean.vi"("X"=w244) -> ("mean"=w238:dbl)  [unwired: 1 out]
              n91 = Array Max & Min(array=w244) -> (max value=w246:dbl, min value=w245:dbl)  [unwired: 2 out]
              n92 = Absolute Value(x=w238) -> (abs(x)=w241:dbl)
              n93 = Subtract(x=w246, y=w245) -> (x-y=w243:dbl)
              n94 = Divide(x=w241, y=95.0) -> (x/y=w239:dbl)
              n95 = Absolute Value(x=w243) -> (abs(x)=w242:dbl)
              n96 = Less?(x=w242, y=w239) -> (x < y?=w237:bool)
            }
            frame #1 {
              n97 = case shown="False" w255 {
                tunnel: w256 -> [w261 _]
                frame False {
                  n98 = Increment(x=w261) -> (x+1=w260:i32)
                  n99 = Format Into String(format string="The positions are not evenly spaced so cannot calculate the spectrum for series %d", w260) -> (resulting string=w258:string)  [unwired: 2 in, 1 out]
                  n100 = One Button Dialog(message=w258, button name ("OK")="stop") -> ()  [unwired: 1 out]
                }
                frame True {
                }
              }
            }
            frame #2 {
              w270 = 2 ("index")
              n101 = Reciprocal(x=w269) -> (1/x=w268:dbl)
              n102 = Array Size(array=w267) -> (size(s)=w271:i32)
              n103 = Divide(x=w268, y=w271) -> (x/y=w265:dbl)
              n104 = call "Power_spectrum.vi"("U"=w267, "Sampling frequency"=w268, "Block No"=1) -> ("SingleBlockSpectrum"=w262:dbl[])  [unwired: 2 in, 2 out]
              n105 = call <vilib>:"Std Deviation and Variance.vi"("X"=w267) -> ("variance"=w266:dbl)  [unwired: 1 in, 2 out]
              n106 = Array Subset(array=w262, index=w270) -> (w264:dbl[])  [unwired: 1 in]
              n107 = Divide(x=w264, y=w266) -> (x/y=w263:dbl[])
              n108 = Array Size(array=w263) -> (size(s)=w274:i32)
              n109 = for {
                N: w274 -> [_]
                tunnel: [w279] -> w273 mode=indexing
                tunnel: w265 -> [w281]
                tunnel: w270 -> [w277]
                i -> [w282]
                n110 = Increment(x=w282) -> (x+1=w278:i32)
                n111 = Add(x=w278, y=w277) -> (x+y=w276:i32)
                n112 = Multiply(x=w276, y=w281) -> (x*y=w280:dbl)
                n113 = Reciprocal(x=w280) -> (1/x=w279:dbl)
              }
              n114 = Bundle(w273, w263) -> (w275:cluster{dbl[], dbl[]})  [unwired: 1 out]
            }
          }
        }
        n115 = And Array Elements(Boolean array=w224) -> (logical AND=w223:bool)
      }
      frame "Do fitting?" {
        n116 = case shown="\"Linear\", Default" w285 {
          tunnel: ["Adjust Plot scales etc" "Poly fit to data"] -> _
          frame "None" {
          }
          frame "Linear", Default {
          }
        }
      }
      frame "Poly fit to data" {
        n117 = case shown="\"None\", Default" w301 {
          tunnel: [0 ("polynomial order") 1 ("polynomial order") 2 ("polynomial order") 3 ("polynomial order") 4 ("polynomial order")] -> w300
          frame "None", Default {
          }
          frame "Linear" {
          }
          frame "2nd Poly" {
          }
          frame "3rd Poly" {
          }
          frame "4th Poly" {
          }
        }
        n118 = for {
          tunnel: w299 -> [w323] mode=indexing
          tunnel: [w324] -> w298 mode=indexing
          tunnel: w300 -> [w322]
          tunnel: [w317] -> w295 mode=indexing
          tunnel: w294 -> [w316]
          tunnel: w293 -> [w315]
          w321 = 8  # Enhancement factor
          n119 = Unbundle(w323) -> ("Output"=w314:dbl[], "PercentageDifferenceArray"=w313:dbl[])
          n120 = call <vilib>:"General Polynomial Fit.vi"("Y"=w313, "polynomial order"=w322, "X"=w314) -> ("Polynomial Coefficients"=w311:dbl[])  [unwired: 9 in, 3 out]
          n121 = case shown="False" "Something about fit..!" {
            tunnel: [w327 w342] -> w318
            tunnel: [w338 w343] -> w317
            tunnel: w316 -> [w340 _]
            tunnel: w315 -> [w339 _]
            tunnel: w314 -> [w335 _]
            tunnel: w313 -> [w332 _]
            tunnel: w311 -> [_ w342]
            frame False {
              w334 = 0.99 ("Voltage")
              n122 = Build Array (concatenate)(nan ("Voltage"), w332) -> (w336:dbl[])
              n123 = Build Array (concatenate)(w334, w335) -> (w337:dbl[])
              n124 = call "Curve_Fit_ph.vi"("Values In"=w336, "No of points to fit (3)"=4, "Positions"=w337) -> ("Values Out"=w331:dbl[], "Polynomial Fit Coefficients"=w327:dbl[])  [unwired: 1 in]
              n125 = Index Array(array=w331, index=0) -> (element=w329:dbl)
              n126 = call "Number_2_string.vi"("precision"="2", "number"=w329) -> ("String"=w325:string)
              n127 = Format Into String(format string="When %s=%.2f ; %s=%s", w340, w334, w339, w325) -> (resulting string=w338:string)  [unwired: 2 in, 1 out]
            }
            frame True {
              n128 = for {
                shift-right: [w345] -> w343
                shift-left: "" -> [w346]
                tunnel: w342 -> [w349] mode=indexing
                i -> [w350]
                n129 = call "Number_2_string.vi"("number"=w349) -> ("String"=w347:string)  [unwired: 1 in]
                n130 = case shown="0, Default" w350 {
                  tunnel: [w351] -> w348
                  tunnel: w347 -> [w353]
                  frame 0, Default {
                    n131 = Concatenate Strings(w353, " ") -> (w351:string)
                  }
                }
                n132 = Concatenate Strings(w346, w348) -> (w345:string)
              }
            }
          }
          n133 = call "Enhance_No_of_points.vi"("Enhancement factor"=w321, "Input"=w314) -> ("Output"=w320:dbl[])  [unwired: 3 out]
          n134 = for {
            tunnel: w318 -> [w356]
            tunnel: w320 -> [w355] mode=indexing
            tunnel: [w354] -> w319 mode=indexing
            n135 = call "Polynomial_convert.vi"("Calib constants"=w356, "Voltage"=w355) -> ("Eng Values"=w354:dbl)  [unwired: 4 out]
          }
          n136 = Bundle("Output"=w320, w319) -> (w324:cluster{"Output":dbl[], dbl[]})  [unwired: 1 out]
        }
        n137 = Build Array (concatenate)(w297, w295) -> (w296:string[])
        n138 = Build Array (concatenate)(w299, w298) -> (w292:T7)
        n139 = local write "XY Graph"(w292) -> ()
      }
      frame "Add fitted line styles" {
        n140 = local read "No of Series"() -> (w357:i32)
        n141 = Array Subset(array=w360, index=w357) -> (w359:string[])  [unwired: 1 in]
        n142 = for {
          tunnel: w359 -> [w368] mode=indexing
          tunnel: u8 2 ("Plot.Plot Interpolation") -> [w374]
          tunnel: w357 -> [w370]
          i -> [w371]
          w376 = u32 0
          n143 = Concatenate Strings(w368, "  " ("string")) -> (w366:string)
          n144 = Add(x=w370, y=w371) -> (x+y=w369:i32)
          n145 = Quotient & Remainder(x=w371, y=4) -> (x-y*floor(x/y)=w372:i32)  [unwired: 1 out]
          n146 = property on="XY Graph" class="XYGraph (strict)"("Active Plot"=w369, "Plot.Plot Name"=w366, "Plot.Fill/Point Color"=w376, "Plot.Plot Color"=w376, "Plot.Point Style"=u8 0, "Plot.Line Style"=w372, "Plot.Plot Interpolation"=w374) -> ()  [unwired: 2 in, 2 out]
        }
      }
      frame "Adjust Plot scales etc" {
        w377 = u8[] [6, 1, 11, 2, 5, 13, 15, 10, 12, 14]  # pointStyles
        n147 = Greater Than 0?(x=w383) -> (x > 0?=w382:bool)
        n148 = Array Size(array=w385) -> (size(s)=w390:i32)
        n149 = local read "No of Series"() -> (w384:i32)
        n150 = property on="XY Graph" class="XYGraph (strict)"("Legend:Plots Shown"=w390) -> ()  [unwired: 2 in, 2 out]
        n151 = case shown="\"None\", Default" w380 {
          tunnel: ["Adjust plot scales2" "Show percentage change" ("t") "Set spectra axis" ("t") "Set spectra axis" ("t")] -> w379
          frame "None", Default {
          }
          frame "% change" {
          }
          frame "Spectrum" {
          }
          frame "Norm Spec" {
          }
        }
        n152 = Select(t=u8 2 ("Plot.Plot Interpolation"), s=w382, f=u8 0 ("Plot.Plot Interpolation")) -> (s? t:f=w386:u8)
        n153 = for {
          N: w384 -> [_]
          tunnel: w385 -> [w404] mode=indexing
          tunnel: w377 -> [w408]
          tunnel: w386 -> [w397]
          i -> [w407]
          w409 = u32 0
          n154 = String Length(string=w404) -> (length=w400:i32)
          n155 = Subtract(x=w400, y=2) -> (x-y=w398:i32)
          n156 = String Subset(string=w404, offset (0)=0, length (rest)=w398) -> (substring=w403:string)
          n157 = Concatenate Strings(w403, "  " ("string")) -> (w401:string)
          n158 = Index Array(array=w408, index=w407) -> (element=w406:u8)
          n159 = property on="XY Graph" class="XYGraph (strict)"("Active Plot"=w407, "Plot.Plot Name"=w401, "Plot.Fill/Point Color"=w409, "Plot.Plot Color"=w409, "Plot.Point Style"=w406, "Plot.Line Style"=u8 0, "Plot.Plot Interpolation"=w397) -> ()  [unwired: 2 in, 2 out]
        }
        "XY Graph" <- w378
      }
      frame "Adjust plot scales2" {
        n160 = property on="XY Graph" class="XYGraph (strict)"("X Scale.Name Label.Text"=w411, "Y Scale.Name Label.Text"=w410, "Cursor.Visible"=FALSE) -> ()  [unwired: 2 in, 2 out]
      }
      frame "Show percentage change" {
        n161 = Concatenate Strings(w422, " % Change" ("string")) -> (w425:string)
        n162 = property on="XY Graph" class="XYGraph (strict)"("X Scale.Name Label.Text"=w423, "Y Scale.Name Label.Text"=w425, "Cursor.Visible"=FALSE) -> ()  [unwired: 2 in, 2 out]
      }
      frame "Set spectra axis" {
        n163 = case shown="\"Spectrum\", Default" w430 {
          tunnel: [" Spectral Energy" ("string") " Normalised Spectral Energy" ("string")] -> w438
          frame "Spectrum", Default {
          }
          frame "Norm Spec" {
          }
        }
        n164 = Concatenate Strings(w435, w438) -> (w437:string)
        n165 = property on="XY Graph" class="XYGraph (strict)"("X Scale.Name Label.Text"="Wavelength [mm]", "Y Scale.Name Label.Text"=w437, "Cursor.Visible"=FALSE) -> ()  [unwired: 2 in, 2 out]
      }
      frame "Fill Second legend" {
        n166 = global read "Results_plotter_Global.vi" "Current Data Filenames"() -> (w448:string)
        n167 = call "Fast_string_Replace.vi"("Replace match with:"="_", "Input String"=w448, "regular expression"="[/]") -> ("Output String"=w452:string)  [unwired: 2 out]
        n168 = call "Fast_string_Replace.vi"("Replace match with:"="_", "Input String"=w452, "regular expression"="__") -> ("Output String"=w449:string)  [unwired: 2 out]
        n169 = call "Fast_string_Replace.vi"("Replace match with:"="", "Input String"=w449, "regular expression"=" ") -> ("Output String"=w447:string)  [unwired: 2 out]
        n170 = String Subset(string=w447, offset (0)=0, length (rest)=30 ("length (rest)")) -> (substring=w446:string)
        n171 = Build Path(base path=w459, name or relative path=w446) -> (appended path=w463:path)
      }
      frame "Calculate plot max and min values" {
        n172 = local read "plot error bars?"() -> (w466:bool)
        n173 = for {
          tunnel: w494 -> [w522] mode=indexing
          shift-right: [w519] -> w490
          shift-left: _ -> [w515]
          shift-right: [w518] -> w491
          shift-left: _ -> [w514]
          shift-right: [w517] -> w485
          shift-left: _ -> [w513]
          shift-right: [w516] -> w484
          shift-left: _ -> [w512]
          tunnel: w467 -> [w510]
          tunnel: w466 -> [w511]
          tunnel: w465 -> [w508]
          i -> [w509]
          n174 = Unbundle(w522) -> ("Output"=w521:dbl[], "PercentageDifferenceArray"=w520:dbl[])
          n175 = case shown="True" w511 {
            tunnel: w510 -> [_ w543]
            tunnel: w509 -> [_ w542]
            tunnel: [0.0 w538] -> w503
            frame False {
            }
            frame True {
              n176 = Index Array(array=w543, index=w542) -> (element=w541:cluster{string[]})
              n177 = Unbundle(w541) -> (w540:string[])
              n178 = Fract/Exp String To Number(string=w540) -> (number=w539:dbl[])  [unwired: 4 out]
              n179 = Array Max & Min(array=w539) -> (max value=w538:dbl)  [unwired: 3 out]
            }
          }
          n180 = Array Max & Min(array=w521) -> (max value=w501:dbl, min value=w499:dbl)  [unwired: 2 out]
          n181 = Array Max & Min(array=w520) -> (max value=w507:dbl, min value=w505:dbl)  [unwired: 2 out]
          n182 = case shown="True" w508 {
            tunnel: w507 -> [w529 w536]
            tunnel: [w528 w536] -> w506
            tunnel: w505 -> [w527 w535]
            tunnel: [w526 w535] -> w504
            tunnel: w503 -> [w525 w534]
            tunnel: [w524 w530] -> w502
            tunnel: w501 -> [w524 w533]
            tunnel: [w523 w531] -> w500
            tunnel: w499 -> [w523 w532]
            frame False {
              n183 = Subtract(x=w527, y=w525) -> (x-y=w526:dbl)
              n184 = Add(x=w529, y=w525) -> (x+y=w528:dbl)
            }
            frame True {
              n185 = Add(x=w533, y=w534) -> (x+y=w530:dbl)
              n186 = Subtract(x=w532, y=w534) -> (x-y=w531:dbl)
            }
          }
          n187 = case shown="1, Default" w509 {
            tunnel: [w547 w561] -> w519
            tunnel: w502 -> [w547 w560]
            tunnel: w500 -> [w546 w557]
            tunnel: [w546 w556] -> w518
            tunnel: [w545 w549] -> w517
            tunnel: w506 -> [w545 w552]
            tunnel: [w544 w548] -> w516
            tunnel: w504 -> [w544 w550]
            tunnel: w515 -> [_ w562]
            tunnel: w514 -> [_ w559]
            tunnel: w513 -> [_ w553]
            tunnel: w512 -> [_ w551]
            frame 0 {
            }
            frame 1, Default {
              n188 = Greater?(x=w553, y=w552) -> (0:w554:bool)
              n189 = Greater?(x=w562, y=w560) -> (0:w563:bool)
              n190 = Less?(x=w551, y=w550) -> (x < y?=w555:bool)
              n191 = Less?(x=w559, y=w557) -> (x < y?=w558:bool)
              n192 = Select(t=w553, s=w554, f=w552) -> (s? t:f=w549:dbl)
              n193 = Select(t=w551, s=w555, f=w550) -> (s? t:f=w548:dbl)
              n194 = Select(t=w562, s=w563, f=w560) -> (s? t:f=w561:dbl)
              n195 = Select(t=w559, s=w558, f=w557) -> (s? t:f=w556:dbl)
            }
          }
        }
        n196 = Subtract(x=w490, y=w491) -> (x-y=w492:dbl)
        n197 = Subtract(x=w485, y=w484) -> (x-y=w487:dbl)
        n198 = Multiply(x=w492, y=0.1) -> (x*y=w489:dbl)
        n199 = Multiply(x=w487, y=0.1) -> (x*y=w488:dbl)
        n200 = Add(x=w490, y=w489) -> (x+y=w477:dbl)
        n201 = Subtract(x=w491, y=w489) -> (x-y=w474:dbl)
        n202 = Add(x=w485, y=w488) -> (x+y=w470:dbl)
        n203 = Subtract(x=w484, y=w488) -> (x-y=w479:dbl)
        n204 = Select(t=w477, s="Xmax", f="Xmax Val") -> (s? t:f=w475:dbl)
        n205 = Select(t=w474, s="Xmin", f="Xmin Val") -> (s? t:f=w482:dbl)
        n206 = Select(t=w470, s="Ymax", f="Ymax Val") -> (s? t:f=w468:dbl)
        n207 = Select(t=w479, s="Ymin", f="Ymin Val") -> (s? t:f=w483:dbl)
        n208 = property on="XY Graph" class="XYGraph (strict)"("X Scale.Range:Maximum"=w475, "X Scale.Range:Minimum"=w482, "Y Scale.Range:Maximum"=w468, "Y Scale.Range:Minimum"=w483) -> ()  [unwired: 2 in, 2 out]
      }
      frame "Sort out plot title" {
        n209 = local read "Summarise"() -> (w577:u16)
        n210 = case shown="1, Default" "Plot Title" {
          selector: "Plot Title" -> [_ w595]
          tunnel: [w594 w601] -> w572
          tunnel: "Plot Title" -> [w594 w600]
          tunnel: w573 -> [_ w604]
          tunnel: w577 -> [_ w598]
          frame 0 {
          }
          frame 1, Default {
            n211 = Decrement(x=w595) -> (x-1=w603:u16)
            n212 = Add(x=w598, y=u16 2) -> (x+y=w597:u16)
            n213 = Index Array(array=w604, index (row)=w603, index (col)=w597) -> (element=w607:string)
            n214 = Empty String/Path?(string/path=w600) -> (empty?=w602:bool)
            n215 = call "Fast_string_Replace.vi"("Replace match with:"="~ ", "Input String"=w607, "regular expression"=":") -> ("Output String"=w606:string)  [unwired: 2 out]
            n216 = call <vilib>:"Trim Whitespace.vi"("string"=w606) -> ("trimmed string"=w605:string)  [unwired: 1 in]
            n217 = call "Fast_string_Replace.vi"("Replace match with:"="~", "Input String"=w605, "regular expression"="_") -> ("Output String"=w596:string)  [unwired: 2 out]
            n218 = case shown="False" w602 {
              tunnel: [w613 w616] -> w601
              tunnel: w596 -> [w615 w616]
              tunnel: w600 -> [w614 _]
              frame False {
                n219 = Concatenate Strings(w614, " " ("string"), w615) -> (w613:string)
              }
              frame True {
              }
            }
          }
        }
        n220 = case shown="False" "Show Labels?" {
          tunnel: w573 -> [w589 _]
          tunnel: w572 -> [w592 w593]
          tunnel: [w590 w593] -> w571
          frame False {
            n221 = local read "Added labels"() -> (w591:i32[])
            n222 = Concatenate Strings(w592, "         " ("string")) -> (w588:string)
            n223 = call "DistillTitle.vi"("Plot Summary in"=w589, "Show Channels with range of Values?"=FALSE, "Indices to include in Page Title"=w591, "String in"=w588) -> ("String out"=w590:string)  [unwired: 6 in, 1 out]
          }
          frame True {
          }
        }
        "Final Title" <- w571
        n224 = Current VI's Path() -> (path=w569:path)
        n225 = call "Running_as_top_level.vi"("Vi path name"=w569) -> ("Top Level"=w567:bool)  [unwired: 1 out]
        n226 = case shown="True" w567 {
          tunnel: [w581 w584] -> w566
          tunnel: w565 -> [w581 _]
          tunnel: ["Get Filename" ("t") "Create plot directory"] -> w564
          frame False {
          }
          frame True {
            n227 = local read "Path"() -> (w583:path)
            n228 = Strip Path(path=w583) -> (name=w582:string)  [unwired: 1 out]
            n229 = Build Path(base path=w583, name or relative path=w582) -> (appended path=w584:path)
          }
        }
      }
      frame "Get Filename" {
        n230 = local read "Final Title"() -> (w620:string)
        n231 = case shown="\"% change\"" w622 {
          tunnel: ["" "Per_" "Spec_" "N_Spec_"] -> w621
          frame "None" {
          }
          frame "% change" {
          }
          frame "Spectrum" {
          }
          frame "Norm Spec" {
          }
        }
        n232 = Concatenate Strings(w621, w620) -> (w617:string)
        n233 = String Length(string=w620) -> (length=w619:i32)
        n234 = case shown="0" w619 {
          tunnel: [w637 w638] -> w618
          tunnel: w617 -> [w637 w640]
          frame 0 {
          }
          frame 1, Default {
            n235 = Concatenate Strings(w640, "_") -> (w638:string)
          }
        }
        n236 = call "Auto_filename.vi"("Filename Max length"="Filename Max length", "Prefix"=w618) -> ("Filename"=w624:string)
        n237 = Build Path(base path=w631, name or relative path=w624) -> (appended path=w628:path)
        n238 = File/Directory Info(path=w628) -> (error out=w629:errorcluster)  [unwired: 1 in, 6 out]
        n239 = Build Path(base path=w628, name or relative path=w624) -> (appended path=w635:path)
        n240 = Unbundle By Name(w629) -> ("status"=w627:bool)
        n241 = Select(t="Create plot directory", s=w627, f="Find a unique name") -> (s? t:f=w634:string)
      }
      frame "Find a unique name" {
        n242 = call "FindUniqueName.vi"("Max Length"=27, "PathIn"=w647) -> ("UniquedPath"=w646:path)  [unwired: 9 in]
      }
      frame "Create plot directory" {
        n243 = Strip Path(path=w655) -> (stripped path=→"Path":path)  [unwired: 1 out]
        n244 = call "Create_directory_path.vi"("Path name"=w655) -> ("Path name Out"=w660:path)  [unwired: 2 in, 1 out]
        n245 = Select(t="Save data analysis file", s="Save data analysis file", f="Save .dat file") -> (s? t:f=w658:string)
      }
      frame "Save data analysis file" {
        n246 = stacked-sequence {
          seq-local: [w675 _ _] -> [_ _ w719]
          seq-local: [_ w691 _] -> [_ _ w717]
          tunnel: w673 -> [_ _ w730]
          tunnel: [_ _ TRUE ("Top Level")] -> w672
          tunnel: [_ _ "Save .dat file"] -> w671
          tunnel: w670 -> [w678 w693 _]
          tunnel: w669 -> [_ _ _]
          tunnel: w668 -> [_ _ _]
          tunnel: w664 -> [_ w694 _]
          tunnel: w666 -> [w682 _ _]
          tunnel: w665 -> [w681 _ _]
          frame #0 {
            n247 = case shown="\"Norm Spec\"" w682 {
              tunnel: w681 -> [w685 w689]
              tunnel: [w684 w688] -> w680
              tunnel: ["Wavelength::[mm]" "Wavelength::[mm]"] -> w679
              frame "Spectrum", Default {
                n248 = Concatenate Strings(w685, ":Spectral:Energy") -> (w684:string)
              }
              frame "Norm Spec" {
                n249 = Concatenate Strings(w689, ":Normalised Spectral:Energy") -> (w688:string)
              }
            }
            n250 = Index Array(array=w678, index (col)=0 ("disabled index (col)")) -> (element=w676:string[])  [unwired: 1 in]
            n251 = Build Array (concatenate)(w679, w680, w676) -> (w675:string[])
          }
          frame #1 {
            n252 = for {
              tunnel: w694 -> [w705] mode=indexing
              tunnel: w693 -> [w702]
              shift-right: [w696] -> w691
              shift-left: string[][] [] -> [w695]
              i -> [w700]
              n253 = Unbundle(w705) -> ("Output"=w704:dbl[], "PercentageDifferenceArray"=w703:dbl[])
              n254 = Add(x=3 ("disabled index (col)"), y=w700) -> (x+y=w699:i32)
              n255 = Index Array(array=w702, index (col)=w699) -> (element=w698:string[])  [unwired: 1 in]
              n256 = for {
                tunnel: w704 -> [w711] mode=indexing
                tunnel: w703 -> [w710] mode=indexing
                tunnel: w698 -> [w707]
                tunnel: [w706] -> w697 mode=indexing
                n257 = call "Number_2_string.vi"("number"=w711) -> ("String"=w709:string)  [unwired: 1 in]
                n258 = call "Number_2_string.vi"("number"=w710) -> ("String"=w708:string)  [unwired: 1 in]
                n259 = Build Array (concatenate)(w709, w708, w707) -> (w706:string[])
              }
              n260 = Build Array (concatenate)(w695, w697) -> (w696:string[][])
            }
          }
          frame #2 {
            w726 = FALSE  # Append last row only
            w725 = FALSE  # exists?
            n261 = Strip Path(path=w730) -> (stripped path=w731:path, name=w733:string)
            n262 = Array Size(array=w717) -> (size(s)=w716:i32[])
            n263 = Concatenate Strings(w733, ".xls" ("string")) -> (w732:string)
            n264 = Index Array(array=w716, index=0) -> (element=w714:i32)
            n265 = Build Path(base path=w731, name or relative path=w732) -> (appended path=w720:path)
            n266 = Initialize Array("", w714) -> (w713:string[])
            n267 = Build Array (concatenate)(w713, w717) -> (w718:string[][])
            n268 = Initialize Array("", 10 ("Dimension Size")) -> (w724:string[])
            n269 = call "Asterisk_header.vi"("Channel names"=w724) -> ("Header string"=w721:string)
            n270 = call "Write_Ch_data_file.vi"("Append last row only"=w726, "Header string"=w721, "exists?"=w725, "Channel Values"=w718, "Channel names"=w719, "Filename"=w720) -> ()  [unwired: 1 in, 5 out]
          }
        }
      }
      frame "Save .dat file" {
        n271 = stacked-sequence {
          seq-local: [w748 _ _ _ _] -> [_ _ _ _ w868]
          seq-local: [_ w774 _ _ _] -> [_ _ _ _ w869]
          seq-local: [_ _ _ w807 _] -> [_ _ _ _ w870]
          seq-local: [_ _ w791 _ _] -> [_ _ _ w805 _]
          seq-local: [_ _ w783 _ _] -> [_ _ _ w802 _]
          seq-local: [_ _ w785 _ _] -> [_ _ _ w801 _]
          tunnel: w746 -> [_ _ _ _ w873]
          tunnel: [_ _ _ _ TRUE ("Top Level")] -> w745
          tunnel: [_ _ _ _ "Gnuplot script Start"] -> w744
          tunnel: w743 -> [w753 _ _ _ _]
          tunnel: w742 -> [_ w777 _ _ _]
          tunnel: w741 -> [_ w773 _ _ _]
          tunnel: w740 -> [_ _ _ w809 _]
          tunnel: w739 -> [_ _ _ w806 _]
          tunnel: w738 -> [_ w771 _ _ _]
          tunnel: [_ _ _ w804 _] -> w737
          tunnel: w736 -> [_ _ w789 _ _]
          tunnel: w735 -> [_ _ _ w803 _]
          tunnel: w734 -> [_ _ w786 _ _]
          frame #0 {
            n272 = Array Subset(array=w753, length (col)=3 ("length")) -> (w751:string[][])  [unwired: 3 in]
            n273 = Build Array("Column Name", "Numeric Tolerance", "Range of Values") -> (w757:string[])
            n274 = Build Array (concatenate)(w757, w751) -> (w749:string[][])
            n275 = for {
              shift-right: [w761] -> w748
              shift-left: "" -> [w758]
              tunnel: w749 -> [w762] mode=indexing
              n276 = for {
                shift-right: [w763] -> w760
                shift-left: w758 -> [w770]
                tunnel: w762 -> [w764] mode=indexing
                i -> [w769]
                n277 = Equal To 0?(x=w769) -> (x = 0?=w768:bool)
                n278 = Select(t="#", s=w768, f="\t") -> (s? t:f=w765:string)
                n279 = Concatenate Strings(w770, w765, w764) -> (w763:string)
              }
              n280 = Concatenate Strings(w760, "\n") -> (w761:string)
            }
          }
          frame #1 {
            w775 = "\n"
            n281 = case shown="\"% change\"" w771 {
              tunnel: w773 -> [w779 w781]
              tunnel: [w779 w780] -> w772
              frame "None", Default {
              }
              frame "% change" {
                n282 = Concatenate Strings(w781, " %" ("string")) -> (w780:string)
              }
            }
            n283 = Concatenate Strings(w775, w775, "#" ("string"), w777, "\t", w772, w775, w775) -> (w774:string)
          }
          frame #2 {
            n284 = global read "Results_plotter_Global.vi" "Precision"() -> (w788:string[])
            n285 = global read "Results_plotter_Global.vi" "Absisca"() -> (w787:i32)
            n286 = case shown="True" "Offset?" {
              tunnel: [0.0 w799] -> w792
              frame False {
              }
              frame True {
                n287 = property on="XY Graph" class="XYGraph (strict)"() -> ("Y Scale.Range:Maximum"=w798:dbl, "Y Scale.Range:Minimum"=w800:dbl)  [unwired: 2 in, 2 out]
                n288 = Subtract(x=w798, y=w800) -> (x-y=w799:dbl)
              }
            }
            "Profile offset" <- w792
            n289 = Index Array(array=w788, index=w787) -> (element=w784:string)
            n290 = case shown="False" w786 {
              tunnel: ["" w796] -> w785
              tunnel: w784 -> [w793 w796]
              tunnel: [w793 ""] -> w783
              frame False {
              }
              frame True {
              }
            }
            n291 = Multiply(x=w792, y=w789) -> (x*y=w791:dbl)
          }
          frame #3 {
            n292 = for {
              tunnel: w809 -> [w836] mode=indexing
              shift-right: [w835] -> w807
              shift-left: "" -> [w826]
              tunnel: w806 -> [w824] mode=indexing
              tunnel: w805 -> [w821]
              tunnel: [w827] -> w804 mode=indexing
              tunnel: w803 -> [w814] mode=indexing
              tunnel: w802 -> [w811]
              tunnel: w801 -> [w810]
              i -> [w831]
              w834 = "\n"
              n293 = Multiply(x=w821, y=w831) -> (x*y=w816:dbl)
              n294 = Unbundle(w836) -> ("Output"=w829:dbl[], "PercentageDifferenceArray"=w830:dbl[])
              n295 = Negate(x=w816) -> (-x=w815:dbl)
              n296 = call "Number_2_string.vi"("number"=w815) -> ("String"=w823:string)  [unwired: 1 in]
              n297 = Format Into String(format string="\\t%s\\tPlot offset", w823) -> (resulting string=w819:string)  [unwired: 2 in, 1 out]
              n298 = Equal To 0?(x=w816) -> (x = 0?=w820:bool)
              n299 = Select(t="", s=w820, f=w819) -> (s? t:f=w817:string)
              n300 = Unbundle(w814) -> (w813:string[])
              n301 = for {
                tunnel: w829 -> [w855] mode=indexing
                shift-right: [w844] -> w833
                shift-left: "" -> [w845]
                tunnel: w830 -> [w852] mode=indexing
                tunnel: w816 -> [w851]
                tunnel: [w850] -> w828 mode=indexing
                tunnel: w813 -> [w847]
                shift-right: [w843] -> _
                shift-left: string[] [] -> [w842]
                tunnel: w811 -> [w839]
                tunnel: w810 -> [w838]
                i -> [w848]
                w849 = "\t"
                n302 = Subtract(x=w852, y=w851) -> (x-y=w850:dbl)
                n303 = call "Number_2_string.vi"("precision"=w839, "number"=w855) -> ("String"=w854:string)
                n304 = call "Number_2_string.vi"("precision"=w838, "number"=w850) -> ("String"=w853:string)
                n305 = Index Array(array=w847, index=w848) -> (element=w846:string)
                n306 = Concatenate Strings(w854, w849, w853, w849, w846, "\n") -> (w841:string)
                n307 = Search 1D Array(1D array=w842, element=w841) -> (index of element=w840:i32)  [unwired: 1 in]
                n308 = case shown="-1" w840 {
                  tunnel: w845 -> [w857 w862]
                  tunnel: [w857 w861] -> w844
                  tunnel: w841 -> [_ w858]
                  tunnel: w842 -> [w856 w860]
                  tunnel: [w856 w859] -> w843
                  frame 0, Default {
                  }
                  frame -1 {
                    n309 = Concatenate Strings(w862, w858) -> (w861:string)
                    n310 = Build Array (concatenate)(w860, w858) -> (w859:string[])
                  }
                }
              }
              n311 = Bundle("Output"=w829, w828) -> (w827:cluster{"Output":dbl[], dbl[]})  [unwired: 1 out]
              n312 = Concatenate Strings(w826, "#", w824, w817, w834, w833, w834, w834) -> (w835:string)
            }
          }
          frame #4 {
            w865 = FALSE  # advisory dialog? (display:T)
            w866 = FALSE  # append to file? (new file:F)
            n313 = Strip Path(path=w873) -> (stripped path=w874:path, name=w876:string)
            n314 = Concatenate Strings(w868, w869, w870) -> (w867:string)
            n315 = Concatenate Strings(w876, ".dat" ("string")) -> (w875:string)
            n316 = Build Path(base path=w874, name or relative path=w875) -> (appended path=w864:path)
            n317 = call "Write_Characters_To_File.vi"("file path (dialog if empty)"=w864, "advisory dialog? (display:T)"=w865, "character string"=w867, "append to file? (new file:F)"=w866) -> ()  [unwired: 1 in, 4 out]
          }
        }
      }
      frame "Gnuplot script Start" {
        n318 = case shown="\"None\", Default" w897 {
          tunnel: w896 -> [w914 w917 w921 w925]
          tunnel: [w914 w916 w920 w924] -> w884
          tunnel: [w913 w915 "Wavelength [mm]" ("X Axis Name") "Wavelength [mm]" ("X Axis Name")] -> w883
          tunnel: w895 -> [w913 w915 _ _]
          frame "None", Default {
          }
          frame "% change" {
            n319 = Concatenate Strings(w917, " % change" ("string")) -> (w916:string)
          }
          frame "Spectrum" {
            n320 = Concatenate Strings(w921, " Spectral energy" ("string")) -> (w920:string)
          }
          frame "Norm Spec" {
            n321 = Concatenate Strings(w925, " Normalised Spectral Energy" ("string")) -> (w924:string)
          }
        }
        n322 = local read "Final Title"() -> (w885:string)
        n323 = case shown="\"Linear\", Default" w889 {
          tunnel: [w904 w906 "Calculate fit parameters"] -> w888
          tunnel: "Edit Legend names" -> [w904 w906 _]
          tunnel: [w903 w905 "set parametric\nset samples 1000\n"] -> w877
          tunnel: "" -> [w903 w905 _]
          frame "None" {
          }
          frame "Spline" {
          }
          frame "Linear", Default {
          }
        }
        n324 = call "setTerm.vi"() -> ("String out"=w882:string)  [unwired: 10 in, 1 out]
        n325 = call "TypesetInsideMathmode.vi"("DirtyString"=w883) -> ("Mathmode String"=w879:string)  [unwired: 8 in, 2 out]
        n326 = call "TypesetInsideMathmode.vi"("DirtyString"=w884) -> ("Mathmode String"=w878:string)  [unwired: 8 in, 2 out]
        n327 = call "TypesetInsideMathmode.vi"("DirtyString"=w885) -> ("Mathmode String"=w881:string)  [unwired: 8 in, 2 out]
        n328 = local read "Time format?"() -> (w890:bool)
        n329 = call "setTitle.vi"("Title"=w881, "String in"=w882) -> ("String out"=w880:string)  [unwired: 8 in, 1 out]
        n330 = Format Into String(format string="set xlabel '%s'\nset ylabel '%s'\nset size %s,%s\n%s", initial string=w880, w879, w878, "Graph width", "Graph Height", w877) -> (resulting string=w892:string)  [unwired: 1 in, 1 out]
        n331 = case shown="True" w890 {
          tunnel: w892 -> [w909 w911]
          tunnel: [w909 w910] -> w891
          frame False {
          }
          frame True {
            n332 = Concatenate Strings(w911, "\nset xdata time\nset timefmt \"%s\"\nset format  x \"%H:%M\\n%Y-%m-%d\"\n") -> (w910:string)
          }
        }
      }
      frame "Calculate fit parameters" {
        # "k=1;    # label 1\nlab=\"23 mA\";\neval( sprintf (\"set label %d %s\", k, lab))"
        n333 = Strip Path(path=w942) -> (name=w941:string)  [unwired: 1 out]
        n334 = Select(t="2:1", s=w931, f="1:2") -> (s? t:f=w932:string)
        n335 = for {
          tunnel: w944 -> [w960]
          tunnel: w941 -> [w958]
          shift-right: [w956] -> w929
          shift-left: w940 -> [w957]
          tunnel: "Auto Zp" -> [w955]
          tunnel: "Fixed Zp" -> [w954]
          tunnel: w932 -> [w953]
          tunnel: w931 -> [w952]
          tunnel: w930 -> [w951] mode=indexing
          tunnel: [w946] -> w927
          i -> [w959]
          n336 = Unbundle(w951) -> ("Output"=w949:dbl[], "PercentageDifferenceArray"=w947:dbl[])
          n337 = case shown="False" w952 {
            tunnel: [w962 w964] -> w950
            tunnel: w949 -> [w962 w963]
            tunnel: [w961 w963] -> w948
            tunnel: w947 -> [w961 w964]
            frame False {
            }
            frame True {
            }
          }
          n338 = case shown="\"Gauss Lat\"" w960 {
            tunnel: w959 -> [w974 w995 w1010 w1029 w1053 w1057 w1063 w1069 _]
            tunnel: w958 -> [w976 w996 w1004 w1034 w1054 w1058 w1064 w1070 _]
            tunnel: w957 -> [w984 w999 w1019 w1044 w1052 w1060 w1066 w1072 w1074]
            tunnel: [w983 w986 w1018 w1043 w1051 w1059 w1065 w1071 w1074] -> w956
            tunnel: w955 -> [_ _ w1009 w1033 _ _ _ _ _]
            tunnel: w954 -> [_ _ w1006 w1030 _ _ _ _ _]
            tunnel: w953 -> [w966 w987 w1003 w1025 w1050 w1056 w1062 w1068 _]
            tunnel: w950 -> [w967 w988 w1002 w1027 _ _ _ _ _]
            tunnel: w948 -> [w968 w989 w1001 w1026 _ _ _ _ _]
            tunnel: [w965 w985 w1000 w1024 w1049 w1055 w1061 w1067 ""] -> w946
            frame "Gauss Lat" {
              w971 = 0.01  # A value of zero make gnuplot stop working
              w965 = "\nf%d(t) = cmax%d*exp(-((t-offset%d)**2)/(2*sig%d**2))\ncmax%d = %.2f; sig%d = %.2f; offset%d = %.2f           # initial guess for cmax and sig and offset\nfit f%d(t) \"%s.dat\" index %d using %s via cmax%d, sig%d, offset%d #this is a gaussian fit\n"
              n339 = Array Max & Min(array=w968) -> (max value=w978:dbl, max index (indices)=w975:i32)  [unwired: 2 out]
              n340 = Array Max & Min(array=w967) -> (max value=w982:dbl, min value=w981:dbl)  [unwired: 2 out]
              n341 = Index Array(array=w967, index=w975) -> (element=w970:dbl)
              n342 = Subtract(x=w982, y=w981) -> (x-y=w980:dbl)
              n343 = Divide(x=w980, y=6.0) -> (x/y=w977:dbl)
              n344 = Absolute Value(x=w970) -> (abs(x)=w972:dbl)
              n345 = Greater?(x=w972, y=w971) -> (0:w973:bool)
              n346 = Select(t=w970, s=w973, f=w971) -> (s? t:f=w969:dbl)
              n347 = Format Into String(format string=w965, initial string=w984, w974, w974, w974, w974, w974, w978, w974, w977, w974, w969, w974, w976, w974, w966, w974, w974, w974) -> (resulting string=w983:string)  [unwired: 1 in, 1 out]
            }
            frame "Guass glc" {
              w992 = 0.01 ("y")
              w985 = "\nf%d(t) = cmax%d*((t/xmax%d)**(-(1+m%d)*q%d)*exp(((1+m%d)/2)*(1-(t/xmax%d)**(-2*q%d))))\ncmax%d = %.2f; xmax%d = %.2f; m%d = 1;  q%d = 0.73         # initial guess for cmax and xmax q and m\nfit f%d(t) \"%s.dat\" index %d using %s via cmax%d, xmax%d, m%d, q%d  #this is a gaussian fit\n"
              n348 = Array Max & Min(array=w989) -> (max value=w998:dbl, max index (indices)=w997:i32)  [unwired: 2 out]
              n349 = Index Array(array=w988, index=w997) -> (element=w991:dbl)
              n350 = Absolute Value(x=w991) -> (abs(x)=w993:dbl)
              n351 = Greater?(x=w993, y=w992) -> (0:w994:bool)
              n352 = Select(t=w991, s=w994, f=w992) -> (s? t:f=w990:dbl)
              n353 = Format Into String(format string=w985, initial string=w999, w995, w995, w995, w995, w995, w995, w995, w995, w995, w998, w995, w990, w995, w995, w995, w996, w995, w987, w995, w995, w995, w995) -> (resulting string=w986:string)  [unwired: 1 in, 1 out]
            }
            frame "Gauss vert" {
              (unwired) "f1(x) = cmax1*exp(-((x-offset1)**2)/(2*sig1**2))"
              w1000 = "\nf%d(t) = cmax%d*(exp(-((t-Zp%d)**2)/(2*sigZ%d**2))+exp(-((t+Zp%d)**2)/(2*sigZ%d**2)))\ncmax%d = %.2f; sigZ%d = %.2f; Zp%d = %.2f           # initial guess for cmax and sig and offset\nfit f%d(t) \"%s.dat\" index %d using %s via cmax%d, sigZ%d%s, Zp%d #this is a gaussian fit\n"
              n354 = Array Max & Min(array=w1001) -> (max value=w1013:dbl, max index (indices)=w1011:i32)  [unwired: 2 out]
              n355 = Array Max & Min(array=w1002) -> (max value=w1017:dbl, min value=w1016:dbl)  [unwired: 2 out]
              n356 = Index Array(array=w1002, index=w1011) -> (element=w1008:dbl)
              n357 = Subtract(x=w1017, y=w1016) -> (x-y=w1015:dbl)
              n358 = Divide(x=w1015, y=6.0) -> (x/y=w1012:dbl)
              n359 = case shown="False" w1009 {
                tunnel: [w1021 w1023] -> w1007
                tunnel: w1008 -> [_ w1023]
                tunnel: w1006 -> [w1021 _]
                tunnel: [" #" ""] -> w1005
                frame False {
                }
                frame True {
                }
              }
              n360 = Format Into String(format string=w1000, initial string=w1019, w1010, w1010, w1010, w1010, w1010, w1010, w1010, w1013, w1010, w1012, w1010, w1007, w1010, w1004, w1010, w1003, w1010, w1010, w1005, w1010) -> (resulting string=w1018:string)  [unwired: 1 in, 1 out]
            }
            frame "Gauss Vert with 2 sig" {
              w1024 = "\nf%d(t) = %s\ncmax%d = %.2f; sigZ_low%d = %.2f; sigZ_up%d = %.2f; Zp%d = %.2f           # initial guess for cmax and sig and offset\nfit f%d(t) \"%s.dat\" index %d using %s via cmax%d, sigZ_low%d, sigZ_up%d%s, Zp%d #this is a gaussian fit\n"
              n361 = Array Max & Min(array=w1026) -> (max value=w1036:dbl, max index (indices)=w1038:i32)  [unwired: 2 out]
              n362 = Array Max & Min(array=w1027) -> (max value=w1042:dbl, min value=w1041:dbl)  [unwired: 2 out]
              n363 = Index Array(array=w1027, index=w1038) -> (element=w1032:dbl)
              n364 = Subtract(x=w1042, y=w1041) -> (x-y=w1040:dbl)
              n365 = Divide(x=w1040, y=6.0) -> (x/y=w1035:dbl)
              n366 = call "Vert_Spread_2_Sig.vi"("Index"=w1029) -> ("resulting string"=w1037:string)
              n367 = case shown="False" w1033 {
                tunnel: [w1046 w1048] -> w1031
                tunnel: w1030 -> [w1046 _]
                tunnel: [" #" ""] -> w1028
                tunnel: w1032 -> [_ w1048]
                frame False {
                }
                frame True {
                }
              }
              n368 = Format Into String(format string=w1024, initial string=w1044, w1029, w1037, w1029, w1036, w1029, w1035, w1029, w1035, w1029, w1031, w1029, w1034, w1029, w1025, w1029, w1029, w1029, w1028, w1029) -> (resulting string=w1043:string)  [unwired: 1 in, 1 out]
            }
            frame "2nd Poly" {
              w1049 = "\nf%d(t) = c%d*t**2 + b%d*t + a%d\n#a%d = 40; b%d = 300; c%d = 1           # initial guess for cmax and sig and offset\nfit f%d(t) \"%s.dat\" index %d using %s via a%d, b%d, c%d #this is a 2nd order poly fit\n"
              n369 = Format Into String(format string=w1049, initial string=w1052, w1053, w1053, w1053, w1053, w1053, w1053, w1053, w1053, w1054, w1053, w1050, w1053, w1053, w1053) -> (resulting string=w1051:string)  [unwired: 1 in, 1 out]
            }
            frame "3rd Poly" {
              w1055 = "\nf%d(t) = d%d*t**3 +c%d*t**2 + b%d*t + a%d\n#a%d = 40; b%d = 300; c%d = 1; d%d = 1         # initial guess for cmax and sig and offset\nfit f%d(t) \"%s.dat\" index %d using %s via a%d, b%d, c%d, d%d #this is a 3rd order poly fit\n"
              n370 = Format Into String(format string=w1055, initial string=w1060, w1057, w1057, w1057, w1057, w1057, w1057, w1057, w1057, w1057, w1057, w1058, w1057, w1056, w1057, w1057, w1057, w1057) -> (resulting string=w1059:string)  [unwired: 1 in, 1 out]
            }
            frame "4th Poly" {
              w1061 = "\nf%d(t) = e%d*t**4 + d%d*t**3 +c%d*t**2 + b%d*t + a%d\n#a%d = 40; b%d = 300; c%d = 1; d%d = 1  e%d = 1       # initial guess for cmax and sig and offset\nfit f%d(t) \"%s.dat\" index %d using %s via a%d, b%d, c%d, d%d, e%d #this is a 3rd order poly fit\n"
              n371 = Format Into String(format string=w1061, initial string=w1066, w1063, w1063, w1063, w1063, w1063, w1063, w1063, w1063, w1063, w1063, w1063, w1063, w1064, w1063, w1062, w1063, w1063, w1063, w1063, w1063) -> (resulting string=w1065:string)  [unwired: 1 in, 1 out]
            }
            frame "Linear" {
              w1067 = "\nf%d(t) = b%d*t + c%d\n#a%d = 40; b%d = 300; c%d = 1           # initial guess for cmax and sig and offset\nfit f%d(t) \"%s.dat\" index %d using %s via b%d, c%d #this is a Linear fit\n"
              n372 = Format Into String(format string=w1067, initial string=w1072, w1069, w1069, w1069, w1069, w1069, w1069, w1069, w1070, w1069, w1068, w1069, w1069) -> (resulting string=w1071:string)  [unwired: 1 in, 1 out]
            }
            frame "Spline", Default {
            }
          }
        }
        n373 = call "ParsingFitFormulae.vi"("String"=w927) -> ("element"=w928:string)
        n374 = local write "Current Fit Formula"(w928) -> ()
        n375 = Concatenate Strings(w929, "save variables 'Coeff.txt'\n") -> (w938:string)
      }
      frame "Edit Legend names" {
        n376 = local read "Profile offset"() -> (w1083:dbl)
        n377 = for {
          tunnel: w1093 -> [w1108] mode=indexing
          tunnel: [w1107] -> w1092 mode=indexing
          tunnel: [w1106] -> w1088
          i -> [w1106]
          n378 = String Length(string=w1108) -> (length=w1111:i32)
          n379 = Subtract(x=w1111, y=2) -> (x-y=w1109:i32)
          n380 = String Subset(string=w1108, length (rest)=w1109) -> (substring=w1101:string)  [unwired: 1 out]
          n381 = Match Pattern(string=w1101, regular expression="=") -> (before substring=w1100:string, match substring=w1099:string, after substring=w1098:string)  [unwired: 2 out]
          n382 = call "Match_Pat_Case_In.vi"("String to match"="legend", "String"=w1100) -> ("offset past match"=w1103:i32)  [unwired: 1 in, 3 out]
          n383 = Greater Than 0?(x=w1103) -> (x > 0?=w1102:bool)
          n384 = case shown="False" w1102 {
            tunnel: [w1112 w1116] -> w1095
            tunnel: w1098 -> [w1113 w1116]
            tunnel: w1100 -> [w1115 _]
            tunnel: w1099 -> [w1114 _]
            frame False {
              n385 = Concatenate Strings(w1115, w1114, w1113) -> (w1112:string)
            }
            frame True {
            }
          }
          n386 = call "Fast_string_Replace.vi"("Replace match with:"=" ", "Input String"=w1095, "regular expression"="_") -> ("Output String"=w1094:string)  [unwired: 2 out]
          n387 = call "Text_for_latex.vi"("Input String"=w1094) -> ("Output String"=w1107:string)
        }
        n388 = Multiply(x=w1085, y=w1083) -> (x*y=w1087:dbl)
        n389 = Decrement(x=w1085) -> (x-1=w1084:dbl)
        n390 = Multiply(x=w1087, y=w1088) -> (x*y=w1082:dbl)
        n391 = Multiply(x=w1083, y=w1084) -> (x*y=w1081:dbl)
        n392 = Add(x=w1081, y=w1082) -> (x+y=→"Extra range":dbl)
        n393 = Equal To 0?(x="Legend Position") -> (x = 0?=w1078:bool)
        n394 = Select(t="Auto Legend Position", s=w1078, f="Specified Legend Position") -> (s? t:f=w1076:string)
      }
      frame "Auto Legend Position" {
        w1120 = T9 {"Appearance"={"layout"="horizontal", "text-sample order"="", "key order"="", "surroundingBox"="", "MaxRows"=0, "MaxCols"=0, "WidthAdjust"=0.0}, "Alignment"={"Horizontal"="center", "Vertical"="bottom"}, "Location"="", "\"At\" location"={"XcoordSys"="", "YcoordSys"="", "Xvalue"=0.0, "Yvalue"=0.0}}  # LegendProperties
        w1118 = "at"  # Location
        # "Don't know if any of this is really required-  maybe for offset plots.....?"
        n395 = property on="XY Graph" class="XYGraph (strict)"() -> ("X Scale.Range:Maximum"=w1129:dbl, "X Scale.Range:Minimum"=w1128:dbl, "Y Scale.Range:Minimum"=w1132:dbl, "Y Scale.Range:Maximum"=w1130:dbl)  [unwired: 2 in, 2 out]
        n396 = local read "Graph Height"() -> (w1140:string)
        n397 = case shown="True" w1135 {
          tunnel: w1129 -> [w1161 w1165]
          tunnel: w1128 -> [w1160 w1164]
          tunnel: [w1161 w1163] -> w1146
          tunnel: [w1160 w1162] -> w1142
          frame False {
          }
          frame True {
            n398 = Logarithm Base 10(1:w1165) -> (0:w1163:dbl)
            n399 = Logarithm Base 10(1:w1164) -> (0:w1162:dbl)
          }
        }
        n400 = case shown="True" w1138 {
          tunnel: w1130 -> [w1167 w1171]
          tunnel: w1132 -> [w1166 w1170]
          tunnel: [w1167 w1169] -> w1153
          tunnel: [w1166 w1168] -> w1131
          frame False {
          }
          frame True {
            n401 = Logarithm Base 10(1:w1170) -> (0:w1168:dbl)
            n402 = Logarithm Base 10(1:w1171) -> (0:w1169:dbl)
          }
        }
        n403 = local read "Extra range"() -> (w1133:dbl)
        n404 = Fract/Exp String To Number(string=w1140) -> (number=w1139:dbl)  [unwired: 4 out]
        n405 = Subtract(x=w1131, y=w1133) -> (x-y=w1152:dbl)
        n406 = Divide(x=0.35 ("y"), y=w1139) -> (x/y=w1151:dbl)
        n407 = Subtract(x=w1153, y=w1152) -> (x-y=w1149:dbl)
        n408 = Subtract(x=w1146, y=w1142) -> (x-y=w1145:dbl)
        n409 = Multiply(x=w1149, y=w1151) -> (x*y=w1155:dbl)
        n410 = Divide(x=w1149, y=10.0) -> (x/y=w1147:dbl)
        "Delta y" <- w1147
        n411 = Multiply(x=0.9 ("y"), y=w1145) -> (x*y=w1156:dbl)
        n412 = Multiply(x=w1145, y=-0.2 ("x")) -> (x*y=w1143:dbl)
        n413 = Subtract(x=w1152, y=w1155) -> (x-y=w1137:dbl)
        n414 = case shown="True" "Show legend?" {
          tunnel: w1137 -> [w1178 w1184]
          tunnel: [w1178 w1182] -> w1126
          tunnel: w1147 -> [_ w1185]
          frame False {
          }
          frame True {
            n415 = local read "No of Series"() -> (w1181:i32)
            n416 = Add(x=0.65, y=w1181) -> (x+y=w1180:dbl)
            n417 = Multiply(x=w1185, y=w1180) -> (x*y=w1183:dbl)
            n418 = Subtract(x=w1184, y=w1183) -> (x-y=w1182:dbl)
          }
        }
        "Y location" <- w1126
        n419 = Add(x=w1156, y=w1142) -> (x+y=w1136:dbl)
        n420 = Add(x=w1142, y=w1143) -> (x+y=→"X location":dbl)
        n421 = case shown="True" w1135 {
          tunnel: w1136 -> [w1172 w1174]
          tunnel: [w1172 w1173] -> w1124
          frame False {
          }
          frame True {
            n422 = Power Of 10(x=w1174) -> (10^x=w1173:dbl)
          }
        }
        n423 = case shown="True" w1138 {
          tunnel: w1137 -> [w1175 w1177]
          tunnel: [w1175 w1176] -> w1123
          frame False {
          }
          frame True {
            n424 = Power Of 10(x=w1177) -> (10^x=w1176:dbl)
          }
        }
        n425 = local read "Appearance"() -> (w1117:T6)
        n426 = Bundle By Name(cluster=w1120, "\"At\" location.Xvalue"=w1124, "\"At\" location.Yvalue"=w1123, "Location"=w1118, "Appearance"=w1117) -> (w1119:T9)
        n427 = call "setKey.vi"("LegendProperties"=w1119, "Set?"="Show legend?", "String in"=w1125) -> ("String out"=w1122:string)  [unwired: 7 in, 1 out]
      }
      frame "Specified Legend Position" {
        w1189 = T9 {"Appearance"={"layout"="horizontal", "text-sample order"="", "key order"="", "surroundingBox"="", "MaxRows"=0, "MaxCols"=0, "WidthAdjust"=0.0}, "Alignment"={"Horizontal"="center", "Vertical"="bottom"}, "Location"="", "\"At\" location"={"XcoordSys"="", "YcoordSys"="", "Xvalue"=0.0, "Yvalue"=0.0}}  # LegendProperties
        # "Not sure if stuff below is required, to provide \"Y location\"?"
        n428 = property on="XY Graph" class="XYGraph (strict)"() -> ("Y Scale.Range:Minimum"=w1199:dbl, "Y Scale.Range:Maximum"=w1197:dbl)  [unwired: 2 in, 2 out]
        n429 = local read "Graph Height"() -> (w1205:string)
        n430 = case shown="True" w1203 {
          tunnel: w1197 -> [w1218 w1222]
          tunnel: w1199 -> [w1217 w1221]
          tunnel: [w1218 w1220] -> w1211
          tunnel: [w1217 w1219] -> w1198
          frame False {
          }
          frame True {
            n431 = Logarithm Base 10(1:w1222) -> (0:w1220:dbl)
            n432 = Logarithm Base 10(1:w1221) -> (0:w1219:dbl)
          }
        }
        n433 = local read "Extra range"() -> (w1200:dbl)
        n434 = local read "Show legend?"() -> (w1190:bool)
        n435 = Fract/Exp String To Number(string=w1205) -> (number=w1204:dbl)  [unwired: 4 out]
        n436 = Subtract(x=w1198, y=w1200) -> (x-y=w1210:dbl)
        n437 = Divide(x=0.35 ("y"), y=w1204) -> (x/y=w1209:dbl)
        n438 = local read "Legend Position"() -> (w1193:u16)
        n439 = Subtract(x=w1211, y=w1210) -> (x-y=w1208:dbl)
        n440 = property on="Legend Position" class="Ring (strict)"() -> ("Strings []"=w1194:string[])  [unwired: 2 in, 2 out]
        n441 = Multiply(x=w1208, y=w1209) -> (x*y=w1213:dbl)
        n442 = Index Array(array=w1194, index=w1193) -> (element=w1187:string)
        n443 = Divide(x=w1208, y=10.0) -> (x/y=w1206:dbl)
        n444 = Subtract(x=w1210, y=w1213) -> (x-y=w1202:dbl)
        n445 = case shown="True" w1190 {
          tunnel: w1202 -> [w1223 w1229]
          tunnel: [w1223 w1227] -> w1195
          tunnel: w1206 -> [_ w1230]
          frame False {
          }
          frame True {
            n446 = local read "No of Series"() -> (w1226:i32)
            n447 = Add(x=0.65, y=w1226) -> (x+y=w1225:dbl)
            n448 = Multiply(x=w1230, y=w1225) -> (x*y=w1228:dbl)
            n449 = Subtract(x=w1229, y=w1228) -> (x-y=w1227:dbl)
          }
        }
        n450 = Bundle By Name(cluster=w1189, "Location"=w1187, "Appearance"="Appearance") -> (w1188:T9)
        n451 = local write "Y location"(w1195) -> ()
        n452 = call "setKey.vi"("LegendProperties"=w1188, "Set?"=w1190, "String in"=w1192) -> ("String out"=w1191:string)  [unwired: 7 in, 1 out]
      }
      frame "Labels?" {
        n453 = call "setAxisGrids.vi"("Minor Gridlines"="Minor Gridlines", "Major Gridlines"="Major Gridlines", "String in"=w1234) -> ("String out"=w1233:string)  [unwired: 7 in, 1 out]
        n454 = Array Size(array="Added labels") -> (size(s)=w1242:i32)
        n455 = local read "Show Labels?"() -> (w1236:bool)
        n456 = Greater Than 0?(x=w1242) -> (x > 0?=w1238:bool)
        n457 = And(x=w1236, y=w1238) -> (x .and. y?=w1237:bool)
        n458 = Select(t="Add Labels to plot", s=w1237, f="Set plot ranges" ("t")) -> (s? t:f=w1239:string)
      }
      frame "Add Labels to plot" {
        n459 = stacked-sequence {
          seq-local: [w1257 _] -> [_ w1302]
          tunnel: [_ w1303] -> w1254
          tunnel: w1253 -> [_ w1304]
          tunnel: [_ "Set plot ranges" ("t")] -> w1250
          tunnel: w1249 -> [w1260 _]
          tunnel: w1248 -> [_ w1299]
          tunnel: w1247 -> [_ w1297]
          frame #0 {
            n460 = local read "Added labels"() -> (w1262:i32[])
            n461 = Index Array(array=w1260, index (col)=0 ("disabled index (col)")) -> (element=w1261:string[])  [unwired: 1 in]
            n462 = for {
              tunnel: w1262 -> [w1287] mode=indexing
              tunnel: w1261 -> [w1292]
              tunnel: w1260 -> [w1291]
              tunnel: "Summarise" -> [w1290]
              shift-right: [w1278] -> w1257
              shift-left: string[] [] -> [w1279]
              n463 = Add(x=w1290, y=u16 2) -> (x+y=w1288:u16)
              n464 = Index Array(array=w1291, index (col)=w1288) -> (element=w1286:string[])  [unwired: 1 in]
              n465 = Index Array(array=w1292, index=w1287) -> (element=w1283:string)
              n466 = Index Array(array=w1286, index=w1287) -> (element=w1277:string)
              n467 = call "Fast_string_Replace.vi"("Replace match with:"=" ", "Input String"=w1283, "regular expression"=":") -> ("Output String"=w1282:string)  [unwired: 2 out]
              n468 = call <vilib>:"Trim Whitespace.vi"("string"=w1282) -> ("trimmed string"=w1281:string)  [unwired: 1 in]
              n469 = Match Pattern(string=w1277, regular expression="=") -> (offset past match=w1275:i32)  [unwired: 4 out]
              n470 = Less Than 0?(x=w1275) -> (x < 0?=w1274:bool)
              n471 = Select(t="%s = %s" ("format string"), s=w1274, f="%s %s" ("format string")) -> (s? t:f=w1271:string)
              n472 = Format Into String(format string=w1271, w1281, w1277) -> (resulting string=w1264:string)  [unwired: 2 in, 1 out]
              n473 = Match Pattern(string=w1264, regular expression=";") -> (offset past match=w1269:i32)  [unwired: 4 out]
              n474 = Match Pattern(string=w1264, regular expression=" to ") -> (offset past match=w1268:i32)  [unwired: 4 out]
              n475 = Less Than 0?(x=w1269) -> (x < 0?=w1266:bool)
              n476 = Less Than 0?(x=w1268) -> (x < 0?=w1267:bool)
              n477 = And(x=w1266, y=w1267) -> (x .and. y?=w1265:bool)
              n478 = case shown="False" w1265 {
                tunnel: w1279 -> [w1293 w1296]
                tunnel: [w1293 w1294] -> w1278
                tunnel: w1264 -> [_ w1295]
                frame False {
                }
                frame True {
                  n479 = Build Array (concatenate)(w1296, w1295) -> (w1294:string[])
                }
              }
            }
          }
          frame #1 {
            n480 = local read "Show legend?"() -> (w1298:bool)
            n481 = local read "X location"() -> (w1301:dbl)
            n482 = local read "Delta y"() -> (w1300:dbl)
            n483 = for {
              shift-right: [w1325] -> w1303
              shift-left: w1304 -> [w1326]
              tunnel: w1302 -> [w1322] mode=indexing
              tunnel: w1301 -> [w1308]
              tunnel: w1300 -> [w1327]
              tunnel: w1299 -> [w1321]
              tunnel: w1298 -> [w1310]
              tunnel: w1297 -> [w1306]
              i -> [w1328]
              n484 = call "Text_for_latex.vi"("Input String"=w1322) -> ("Output String"=w1316:string)
              n485 = case shown="False" w1306 {
                tunnel: w1308 -> [w1331 w1333]
                tunnel: [w1331 w1332] -> w1307
                frame False {
                }
                frame True {
                  n486 = Power Of 10(x=w1333) -> (10^x=w1332:dbl)
                }
              }
              n487 = String Length(string=w1316) -> (length=w1319:i32)
              n488 = Less?(x=w1319, y=20) -> (x < y?=w1311:bool)
              n489 = Compound Arithmetic op=AND(w1311, invert w1310) -> (w1309:bool)
              n490 = Increment(x=w1328) -> (x+1=w1329:i32)
              n491 = case shown="True" w1309 {
                tunnel: [w1334 w1336] -> w1317
                tunnel: w1316 -> [w1334 w1337]
                tunnel: "~~~~~~~~~~~" -> [_ w1335]
                frame False {
                }
                frame True {
                  n492 = Concatenate Strings(w1335, w1337) -> (w1336:string)
                }
              }
              n493 = Multiply(x=w1328, y=w1327) -> (x*y=w1323:dbl)
              n494 = local read "Y location"() -> (w1324:dbl)
              n495 = call "Number_2_string.vi"("number"=w1307) -> ("String"=w1314:string)  [unwired: 1 in]
              n496 = Subtract(x=w1324, y=w1323) -> (x-y=w1320:dbl)
              n497 = case shown="False" w1321 {
                tunnel: w1320 -> [w1338 w1340]
                tunnel: [w1338 w1339] -> w1313
                frame False {
                }
                frame True {
                  n498 = Power Of 10(x=w1340) -> (10^x=w1339:dbl)
                }
              }
              n499 = call "Number_2_string.vi"("number"=w1313) -> ("String"=w1312:string)  [unwired: 1 in]
              n500 = Format Into String(format string="set label %d '%s' at %s, %s\n", initial string=w1326, w1329, w1317, w1314, w1312) -> (resulting string=w1325:string)  [unwired: 1 in, 1 out]
            }
          }
        }
      }
      frame "Set plot ranges" {
        w1341 = ""
        (unwired) "set border"
        (unwired) "set nologscale  y"
        (unwired) "set logscale  y"
        w1343 = "#"
        w1345 = ""
        n501 = local read "Profile offset"() -> (w1368:dbl)
        n502 = property on="XY Graph" class="XYGraph (strict)"() -> ("X Scale.Range:Maximum"=w1378:dbl, "X Scale.Range:Minimum"=w1377:dbl, "Y Scale.Range:Maximum"=w1361:dbl, "Y Scale.Range:Minimum"=w1362:dbl)  [unwired: 2 in, 2 out]
        n503 = local read "Extra range"() -> (w1372:dbl)
        n504 = Decrement(x=w1367) -> (x-1=w1369:dbl)
        n505 = Multiply(x=w1368, y=w1369) -> (x*y=w1366:dbl)
        n506 = Add(x=w1366, y=w1361) -> (x+y=w1365:dbl)
        n507 = Subtract(x=w1362, y=w1372) -> (x-y=w1373:dbl)
        n508 = call "Number_2_string.vi"("number"=w1365) -> ("String"=w1350:string)  [unwired: 1 in]
        n509 = call "Gnuplot_offset_ytics.vi"("Separation"=w1367, "Mode"="Mode", "precision"="precision", "Legend"=w1370, "Max Plot Value"=w1361, "Profile offset"=w1368) -> ("concatenated string"=w1357:string)
        n510 = call "Number_2_string.vi"("number"=w1378) -> ("String"=w1352:string)  [unwired: 1 in]
        n511 = call "Number_2_string.vi"("number"=w1377) -> ("String"=w1353:string)  [unwired: 1 in]
        n512 = call "Number_2_string.vi"("number"=w1373) -> ("String"=w1351:string)  [unwired: 1 in]
        n513 = case shown="True" w1354 {
          tunnel: [w1390 w1392] -> w1348
          tunnel: w1353 -> [w1390 _]
          tunnel: [w1389 w1391] -> w1347
          tunnel: w1352 -> [w1389 _]
          tunnel: w1351 -> [_ w1392]
          tunnel: w1350 -> [_ w1391]
          frame False {
          }
          frame True {
          }
        }
        n514 = local read "Time format?"() -> (w1342:bool)
        n515 = Select(t="\nset logscale  x\n", s=w1359, f=w1345) -> (s? t:f=w1356:string)
        n516 = Select(t="\nset logscale  y\n", s=w1364, f=w1345) -> (s? t:f=w1358:string)
        n517 = case shown="\"Linear\", Default" w1349 {
          tunnel: w1348 -> [_ w1387]
          tunnel: w1347 -> [_ w1386]
          tunnel: ["" w1385] -> w1346
          frame "Spline" {
          }
          frame "Linear", Default {
            n518 = Format Into String(format string="set trange [%s : %s]", w1387, w1386) -> (resulting string=w1385:string)  [unwired: 2 in, 1 out]
          }
        }
        n519 = Select(t=w1341, s=w1342, f=w1343) -> (s? t:f=w1344:string)
        n520 = Format Into String(format string="%s set xrange [%s : %s] \n%s set autoscale x \n%s set yrange [%s : %s]\n%s set autoscale y\n", initial string=w1380, w1341, w1353, w1352, w1344, w1341, w1351, w1350, w1343) -> (resulting string=w1375:string)  [unwired: 1 in, 1 out]
        n521 = Concatenate Strings(w1375, w1346, w1356, w1358, w1357) -> (w1376:string)
      }
      frame "Plot Command" {
        n522 = case shown="True" w1402 {
          tunnel: ["yerrorbars" "xerrorbars"] -> w1401
          tunnel: ["" ", t"] -> w1400
          tunnel: ["t, " ""] -> w1399
          frame False {
          }
          frame True {
          }
        }
        n523 = Strip Path(path=w1414) -> (name=w1396:string)  [unwired: 1 out]
        n524 = Format Into String(format string="\nfile=\"%s.dat\"\n\nplot ", w1396) -> (resulting string=w1397:string)  [unwired: 2 in, 1 out]
        n525 = global read "Results_plotter_Global.vi" "Series Index"() -> (w1403:i32[])
        n526 = for {
          shift-right: [w1460] -> w1395
          shift-left: w1397 -> [w1461]
          tunnel: w1408 -> [w1459]
          tunnel: w1413 -> [w1454] mode=indexing
          tunnel: "Plot style" -> [w1455]
          tunnel: w1406 -> [w1442]
          tunnel: w1405 -> [w1453] mode=indexing
          tunnel: "plot error bars?" -> [w1449]
          tunnel: w1401 -> [w1433]
          tunnel: w1403 -> [w1426] mode=indexing
          tunnel: w1400 -> [w1429]
          tunnel: w1399 -> [w1428]
          tunnel: "Fit Line Width" -> [w1422]
          i -> [w1430]
          n527 = Index Array(array=w1455, index=w1426) -> (element=w1437:u16)
          n528 = Quotient & Remainder(x=w1426, y=8) -> (x-y*floor(x/y)=w1441:i32)  [unwired: 1 out]
          n529 = call "Fast_string_Replace.vi"("Replace match with:"="", "Input String"=w1454, "regular expression"="[$]") -> ("Output String"=w1444:string)  [unwired: 2 out]
          n530 = case shown="2" w1437 {
            tunnel: ["points" ("format string") "lines" ("format string") "linespoints" ("format string")] -> w1434
            frame 0, Default {
            }
            frame 1 {
            }
            frame 2 {
            }
          }
          n531 = case shown="\"Spline\"" w1459 {
            tunnel: w1430 -> [_ w1472 w1479 w1486 w1493 w1501 w1508 w1515 w1522 w1529]
            tunnel: ["" w1473 w1480 w1487 w1495 w1502 w1509 w1516 w1523 w1530] -> w1458
            tunnel: w1426 -> [_ w1471 w1478 w1484 w1492 w1500 w1507 w1514 w1521 w1528]
            tunnel: "Fit Line Type" -> [_ w1470 w1477 w1485 w1491 w1499 w1506 w1513 w1520 w1527]
            tunnel: w1429 -> [_ _ w1475 w1483 w1489 w1497 w1504 w1511 w1518 w1525]
            tunnel: w1428 -> [_ _ w1476 w1482 w1490 w1498 w1505 w1512 w1519 w1526]
            tunnel: w1422 -> [_ w1469 _ _ _ _ _ _ _ _]
            frame "None", Default {
            }
            frame "Spline" {
              n532 = Format Into String(format string="file index %d using 1:2 axes x1y1 title'' linecolor %d lw %d linetype %d  smooth csplines, ", w1472, w1471, w1469, w1470) -> (resulting string=w1473:string)  [unwired: 2 in, 1 out]
            }
            frame "Gauss Lat" {
              n533 = Format Into String(format string="%s cmax%d*exp(-((t-offset%d)**2)/(2*sig%d**2))%s  linecolor %d linetype %d title '', ", w1476, w1479, w1479, w1479, w1475, w1478, w1477) -> (resulting string=w1480:string)  [unwired: 2 in, 1 out]
            }
            frame "Gauss vert" {
              n534 = Format Into String(format string="%s cmax%d*(exp(-((t-Zp%d)**2)/(2*sigZ%d**2))+exp(-((t+Zp%d)**2)/(2*sigZ%d**2)))%s linecolor %d linetype %d title '', ", w1482, w1486, w1486, w1486, w1486, w1486, w1483, w1484, w1485) -> (resulting string=w1487:string)  [unwired: 2 in, 1 out]
            }
            frame "Gauss Vert with 2 sig" {
              n535 = call "Vert_Spread_2_Sig.vi"("Index"=w1493) -> ("resulting string"=w1494:string)
              n536 = Format Into String(format string="%s %s%s  linecolor %d linetype %d title '', ", w1490, w1494, w1489, w1492, w1491) -> (resulting string=w1495:string)  [unwired: 2 in, 1 out]
            }
            frame "Guass glc" {
              n537 = Format Into String(format string="%s cmax%d*((t/xmax%d)**(-(1+m%d)*q%d)*exp(((1+m%d)/2)*(1-(t/xmax%d)**(-2*q%d))))%s  linecolor %d linetype %d title '', ", w1498, w1501, w1501, w1501, w1501, w1501, w1501, w1501, w1497, w1500, w1499) -> (resulting string=w1502:string)  [unwired: 2 in, 1 out]
            }
            frame "2nd Poly" {
              n538 = Format Into String(format string="%s c%d*t**2 + b%d*t + a%d%s  linecolor %d linetype %d title 'fit%d', ", w1505, w1508, w1508, w1508, w1504, w1507, w1506, w1508) -> (resulting string=w1509:string)  [unwired: 2 in, 1 out]
            }
            frame "3rd Poly" {
              n539 = Format Into String(format string="%s d%d*t**3  + c%d*t**2 + b%d*t + a%d %s linecolor %d linetype %d title 'fit%d', ", w1512, w1515, w1515, w1515, w1515, w1511, w1514, w1513, w1515) -> (resulting string=w1516:string)  [unwired: 2 in, 1 out]
            }
            frame "4th Poly" {
              n540 = Format Into String(format string="%s e%d*t**4 + d%d*t**3  + c%d*t**2 + b%d*t + a%d%s  linecolor %d linetype %d title 'fit%d', ", w1519, w1522, w1522, w1522, w1522, w1522, w1518, w1521, w1520, w1522) -> (resulting string=w1523:string)  [unwired: 2 in, 1 out]
            }
            frame "Linear" {
              n541 = Format Into String(format string="%s b%d*t + c%d%s  linecolor %d linetype %d title 'fit%d', ", w1526, w1529, w1529, w1525, w1528, w1527, w1529) -> (resulting string=w1530:string)  [unwired: 2 in, 1 out]
            }
          }
          n542 = Index Array(array=w1442, index=w1441) -> (element=w1424:i32)
          n543 = case shown="True" "Black and white?" {
            tunnel: w1426 -> [w1463 _]
            tunnel: [w1463 0] -> w1425
            frame False {
            }
            frame True {
            }
          }
          n544 = Unbundle(w1453) -> (w1452:string[])
          n545 = Array Size(array=w1452) -> (size(s)=w1451:i32)
          n546 = Greater Than 0?(x=w1451) -> (x > 0?=w1450:bool)
          n547 = And(x=w1450, y=w1449) -> (x .and. y?=w1435:bool)
          n548 = Select(t=w1433, s=w1435, f=w1434) -> (s? t:f=w1432:string)
          n549 = Select(t=":3", s=w1435, f="") -> (s? t:f=w1445:string)
          n550 = Format Into String(format string="file index %d using 1:2%s axes x1y1 title '$%s$' with ", initial string=w1461, w1430, w1445, w1444) -> (resulting string=w1448:string)  [unwired: 1 in, 1 out]
          n551 = Format Into String(format string=" linecolor %d pointtype %d pointsize %.2f linetype %d, ", initial string=w1432, w1425, w1424, "Point Size", w1424) -> (resulting string=w1436:string)  [unwired: 1 in, 1 out]
          n552 = Concatenate Strings(w1448, w1436, w1458, "\\" ("string"), "\n") -> (w1460:string)
        }
        n553 = call "removeLastContinuation.vi"("String in"=w1395) -> ("String out"=w1394:string)  [unwired: 10 in]
        n554 = Concatenate Strings(w1412, w1394) -> (w1411:string)
      }
      frame "Write gnuplot file" {
        w1540 = FALSE  # append to file? (new file:F)
        w1541 = FALSE  # advisory dialog? (display:T)
        n555 = Strip Path(path=w1537) -> (stripped path=w1533:path)  [unwired: 1 out]
        n556 = Build Path(base path=w1533, name or relative path="gnuplot_script.txt") -> (appended path=w1542:path)
        n557 = call "gnuplot_legend.vi"("Plot style"=w1534, "Legend"=w1538) -> ()  [unwired: 1 out]
        n558 = call "Write_Characters_To_File.vi"("file path (dialog if empty)"=w1542, "advisory dialog? (display:T)"=w1541, "character string"=w1532, "append to file? (new file:F)"=w1540) -> ()  [unwired: 1 in, 4 out]
      }
      frame "Execute shell script" {
        n559 = call "Run_Gnuplot_Script.vi"("logfileName"=w1544, "workingDirectory"=w1545) -> ()  [unwired: 1 in]
      }
      frame "Has pdf been generated?" {
        n560 = Strip Path(path=w1558) -> (stripped path=w1560:path, name=w1562:string)
        n561 = Concatenate Strings(w1562, ".pdf" ("string")) -> (w1561:string)
        n562 = Build Path(base path=w1560, name or relative path=w1561) -> (appended path=w1557:path)
        n563 = call "Does_file_exist_(simple).vi"("Pathname"=w1557) -> ("exists?"=w1556:bool)
        n564 = case shown="False" w1556 {
          tunnel: ["Open Standard output file" ("f") "Input Fit Coefficients into results file?"] -> w1551
          frame False {
          }
          frame True {
          }
        }
        n565 = Select(t="Show Re-Run Gnuplot?", s="Show Re-Run Gnuplot?", f=w1551) -> (s? t:f=w1552:string)
      }
      frame "Show Re-Run Gnuplot?" {
        n566 = Strip Path(path=w1569) -> (stripped path=w1568:path)  [unwired: 1 out]
        n567 = call "Re_run_Gnuplot.vi"("Plot folder (dialog if empty)"=w1568) -> ()  [unwired: 1 in, 3 out]
      }
      frame "Input Fit Coefficients into results file?" {
        n568 = Greater?(x=w1579, y=T4."Spline" ("Fit type")) -> (0:w1578:bool)
        n569 = And(x="Put Coeff\nin Results file", y=w1578) -> (x .and. y?=w1576:bool)
      }
      frame "Read Fit Coefficients" {
        n570 = call "Fast_string_Replace.vi"("Replace match with:"="", "Input String"=w1586, "regular expression"=":") -> ("Output String"=w1585:string)  [unwired: 2 out]
        n571 = Strip Path(path=w1598) -> (stripped path=w1596:path)  [unwired: 1 out]
        n572 = Build Path(base path=w1596, name or relative path="Coeff.txt") -> (appended path=w1595:path)
        n573 = call "Read_File_Simple.vi"("Filename"=w1595) -> ("string"=w1593:string)  [unwired: 2 in, 7 out]
        n574 = for {
          tunnel: w1594 -> [w1622]
          tunnel: w1593 -> [w1621]
          tunnel: [w1611] -> w1592
          tunnel: w1591 -> [w1619] mode=indexing
          shift-right: [w1616] -> w1589
          shift-left: string[][] [] -> [w1617]
          tunnel: w1585 -> [w1603]
          i -> [w1613]
          n575 = case shown="\"Gauss Lat\"" w1622 {
            tunnel: w1613 -> [_ w1648 w1661 w1672 w1676 w1693 w1707]
            tunnel: [string[] [] w1644 w1657 w1669 w1684 w1699 w1711] -> w1610
            tunnel: [string[] [] w1640 w1653 w1666 w1681 w1696 w1710] -> w1620
            frame "None", Default {
            }
            frame "Gauss Lat" {
              n576 = Format Into String(format string="sig%d", w1648) -> (resulting string=w1646:string)  [unwired: 2 in, 1 out]
              n577 = Format Into String(format string="offset%d", w1648) -> (resulting string=w1645:string)  [unwired: 2 in, 1 out]
              n578 = Format Into String(format string="cmax%d", w1648) -> (resulting string=w1647:string)  [unwired: 2 in, 1 out]
              n579 = Build Array(":Max:Lat", ":Sig Y:", ":Yo:", ":FitFormula:Lat") -> (w1640:string[])
              n580 = Build Array(w1647, w1646, w1645) -> (w1644:string[])
            }
            frame "2nd Poly" {
              n581 = Format Into String(format string="b%d", w1661) -> (resulting string=w1659:string)  [unwired: 2 in, 1 out]
              n582 = Format Into String(format string="c%d", w1661) -> (resulting string=w1658:string)  [unwired: 2 in, 1 out]
              n583 = Format Into String(format string="a%d", w1661) -> (resulting string=w1660:string)  [unwired: 2 in, 1 out]
              n584 = Build Array(":Coeff:A", ":Coeff:B", ":Coeff:C", ":FitFormula:Poly2") -> (w1653:string[])
              n585 = Build Array(w1660, w1659, w1658) -> (w1657:string[])
            }
            frame "Linear" {
              n586 = Format Into String(format string="c%d", w1672) -> (resulting string=w1671:string)  [unwired: 2 in, 1 out]
              n587 = Format Into String(format string="b%d", w1672) -> (resulting string=w1670:string)  [unwired: 2 in, 1 out]
              n588 = Build Array(":Offset:A", ":Grad:B", ":FitFormula:Lin") -> (w1666:string[])
              n589 = Build Array(w1671, w1670) -> (w1669:string[])
            }
            frame "Gauss Vert with 2 sig" {
              n590 = Format Into String(format string="Zp%d", w1676) -> (resulting string=w1685:string)  [unwired: 2 in, 1 out]
              n591 = Format Into String(format string="cmax%d", w1676) -> (resulting string=w1687:string)  [unwired: 2 in, 1 out]
              n592 = Format Into String(format string="sigZ_low%d", w1676) -> (resulting string=w1677:string)  [unwired: 2 in, 1 out]
              n593 = Format Into String(format string="sigZ_up%d", w1676) -> (resulting string=w1686:string)  [unwired: 2 in, 1 out]
              n594 = Build Array(":Max:Vert", ":Sig Z:Upper", ":Sig Z:Lower", ":Zp:", ":FitFormula:Vert2sig") -> (w1681:string[])
              n595 = Build Array(w1687, w1686, w1677, w1685) -> (w1684:string[])
            }
            frame "Gauss vert" {
              n596 = Format Into String(format string="Zp%d", w1693) -> (resulting string=w1700:string)  [unwired: 2 in, 1 out]
              n597 = Format Into String(format string="cmax%d", w1693) -> (resulting string=w1701:string)  [unwired: 2 in, 1 out]
              n598 = Format Into String(format string="sigZ%d", w1693) -> (resulting string=w1692:string)  [unwired: 2 in, 1 out]
              n599 = Build Array(":Max:Vert", ":Sig Z:Upper", ":Sig Z:Lower", ":Zp:", ":FitFormula:Vert") -> (w1696:string[])
              n600 = Build Array(w1701, w1692, w1692, w1700) -> (w1699:string[])
            }
            frame "Guass glc" {
              n601 = Format Into String(format string="xmax%d", w1707) -> (resulting string=w1716:string)  [unwired: 2 in, 1 out]
              n602 = Format Into String(format string="m%d", w1707) -> (resulting string=w1715:string)  [unwired: 2 in, 1 out]
              n603 = Format Into String(format string="q%d", w1707) -> (resulting string=w1706:string)  [unwired: 2 in, 1 out]
              n604 = Format Into String(format string="cmax%d", w1707) -> (resulting string=w1717:string)  [unwired: 2 in, 1 out]
              n605 = Build Array(":MaxC:glc", ":MaxX:glc", ":m:glc", ":q:glc", ":FitFormula:glc") -> (w1710:string[])
              n606 = Build Array(w1717, w1716, w1715, w1706) -> (w1711:string[])
            }
          }
          n607 = global read "Results_plotter_Global.vi" "Full Ch Names"() -> (w1605:string[])
          n608 = global read "Results_plotter_Global.vi" "Absisca"() -> (w1606:i32)
          n609 = Index Array(array=w1605, index=w1606) -> (element=w1604:string)
          n610 = for {
            tunnel: w1603 -> [w1630]
            tunnel: w1620 -> [w1629] mode=indexing
            tunnel: [w1628] -> w1611 mode=indexing
            n611 = Concatenate Strings(w1630, w1629) -> (w1628:string)
          }
          n612 = Unbundle(w1619) -> ("Output"=w1614:dbl[])  [unwired: 1 out]
          n613 = Array Size(array=w1614) -> (size(s)=w1615:i32)
          n614 = for {
            tunnel: w1610 -> [w1636] mode=indexing
            tunnel: w1621 -> [w1633]
            tunnel: [w1631] -> w1609 mode=indexing
            n615 = Concatenate Strings(w1636, " = " ("string")) -> (w1634:string)
            n616 = Match Pattern(string=w1633, regular expression=w1634) -> (after substring=w1632:string)  [unwired: 4 out]
            n617 = call "Split_at_return.vi"("String"=w1632) -> ("before substring"=w1631:string)  [unwired: 1 in, 3 out]
          }
          n618 = call "ReformatFitFormula.vi"("Current Fit Formula"="Current Fit Formula", "Curve Fit Index"=w1613, "Variables"=w1610, "Channel Names"=w1611, "X Axis Full Ch Name"=w1604) -> ("Reformatted Current Fit Formula"=w1608:string)
          n619 = disable-structure shown="Enabled" {
            disable-tunnel: w1609 -> [w1625 w1626]
            disable-tunnel: w1608 -> [w1624 _]
            disable-tunnel: [w1623 w1626] -> w1607
            frame Enabled {
              n620 = Build Array (concatenate)(w1625, w1624) -> (w1623:string[])
            }
            frame Disabled {
            }
          }
          n621 = for {
            N: w1615 -> [_]
            tunnel: w1607 -> [w1627]
            tunnel: [w1627] -> w1618 mode=indexing
          }
          n622 = Build Array (concatenate)(w1617, w1618) -> (w1616:string[][])
        }
        n623 = global write "Results_plotter_Global.vi" "New Chs In"(w1592) -> ()
        n624 = global write "Results_plotter_Global.vi" "New Values In"(w1589) -> ()
      }
      frame "Open Standard output file" {
        n625 = Strip Path(path=w1725) -> (stripped path=w1722:path)  [unwired: 1 out]
        n626 = Format Into String(format string="open \"%s\"", w1723) -> (resulting string=w1721:string)  [unwired: 2 in, 1 out]
        n627 = call <vilib>:"System Exec.vi"("working directory"=w1722, "command line"=w1721) -> ()  [unwired: 4 in, 6 out]
      }
    }
  }
  "Tex Info String" <- w17
  "Saved Automatically?" <- FALSE
